vi "Dust_Source_Control.vi"(7 "error in":errorcluster) -> (0 "error out":errorcluster)   [LabVIEW 2015]
doc: "This VI specifies the properties of the pulse used for running the dust source. When program is stopped, the voltage is incrementally reduced to zero to avoid quick drops."
uses:
  Controls/dust_source_control.ctl
  Controls/XYVoltageFGV.ctl
  <vilib>/Utility/miscctls.llb/LVPointTypeDef.ctl
  <vilib>/Utility/error.llb/DialogType.ctl
  <vilib>/Utility/miscctls.llb/LVMinMaxIncTypeDef.ctl
  <vilib>/Utility/miscctls.llb/LVRangeTypeDef.ctl
  <vilib>/DAQmx/read.llb/DAQmx Read (Analog 1D Wfm NChan NSamp).vi
  <vilib>/Analysis/baseanly.llb/Mean (DBL).vi
  <vilib>/DAQmx/write.llb/DAQmx Write (Analog 1D Wfm NChan NSamp).vi
  <vilib>/DAQmx/read.llb/DAQmx Read (Counter U32 1Chan 1Samp).vi
  <vilib>/DAQmx/create/channels.llb/DAQmx Create Channel (AI-Voltage-Basic).vi
  <vilib>/DAQmx/configure/timing.llb/DAQmx Timing (Sample Clock).vi
  <vilib>/DAQmx/miscellaneous.llb/DAQmx Fill In Error Info.vi
  <vilib>/measure/mascope.llb/Amplitude and Levels 1 chan.vi
  <vilib>/DAQmx/create/channels.llb/DAQmx Create Channel (AO-Voltage-Basic).vi
  Global Variables/throttle.vi
  <userlib>/_OpenG.lib/comparison/comparison.llb/Boolean Changed__ogtk.vi
  Global Variables/throttle from query.vi
  <userlib>/_OpenG.lib/comparison/comparison.llb/DBL Changed__ogtk.vi
  Sub-Polymorphic/post_run_times.vi
  <vilib>/DAQmx/create/channels.llb/DAQmx Create Channel (CI-Count Edges).vi
  Sub-Polymorphic/update_counter_entry_big.vi
  Sub-Polymorphic/post_dust_source.vi
  <vilib>/addons/database/_DB Variant To Data/Database Variant To Data.xnode
  <resource>/objmgr/daqmx.rc
  <vilib>/measure/NI_MAPro.lvlib
  <vilib>/Analysis/NI_AALBase.lvlib
panel:
  out "Einzel and Steering":T1
  out "Y Vs":dbl[](array[numeric])
  out "X Vs":dbl[](array[numeric])
  out "Einzel Vs":dbl[](array[numeric])
  out "Old Einzel":dbl min=0.0 max=10.0 step=0.01 format="%.2g"
  out "Rate Data":dbl[][][](array[numeric])
  out "Freq. Before Throttle":dbl
  out "On/Off":bool
  out "Finished":bool=TRUE
  out "Output waveform":waveform(dbl)={"t0"=timestamp(0 s since 1904-01-01), "dt"=4e-06, "Y"=array[50000 elements]}
  out "Input waveform":waveform(dbl)={"t0"=timestamp(3437998856.0330505 s since 1904-01-01), "dt"=0.00019999999999999998, "Y"=array[1000 elements], "attributes"=variant("NI_ChannelName"=variant(string "Dev5/ai20"), "NI_UnitDescription"=variant(string "Volts"))}
  out "output cluster":T2={"Integer Timestamp"=0, "Einzel Voltage"=0.0, "Needle Voltage"=0.0, "Frequency"=1.0, "Width (ms) : 0.1 "=0.1, "Desired Amplitude (V)"=0.0, "X Voltage"=0.0, "Y Voltage"=0.0, "Settings ID"="", "ID#"=0} {"Needle Voltage" min=0.0 max=10.0 step=0.01 format="%.2g"; "Y Voltage" min=0.0 max=9.0 step=0.01 format="%.2g"; "X Voltage" min=0.0 max=9.0 step=0.01 format="%.2g"; "Einzel Voltage" min=0.0 max=10.0 step=0.01 format="%.2g"; "Desired Amplitude (V)" min=0.0 max=10.0 step=0.01 format="%5.2f"; "Width (ms) : 0.1" min=0.05 max=5.0 step=0.01 format="%6.2f"; "Frequency" min=1.0 max=100.0 step=0.01 format="%.1f"}
  in  "Tab Control":T3(tab)
  out "Current":dbl format="%.2f"
  out "Actual output width (ms)":dbl caption="Output Width (ms)" format="%.2f"
  out "Actual output Frequency":dbl caption="Output  Freq.(hz)" format="%.2f"
  in  "Width (ms) : 0.1":dbl=0.1 caption="Width (ms)" min=0.0 max=5.0 step=0.01 format="%6.2f"
  out "Tube Drive":dbl=0.0012999050305587314 format="%.2f"
  in  "Desired Amplitude (V)":dbl caption="Amplitude (V)" min=0.0 max=10.0 step=0.01 format="%5.2f"
  out "Actual output Amplitude (V)":dbl caption="Output Amp. (V)" format="%.2f"
  in  "Frequency":dbl=1.0 caption="Freq. (Hz)" min=0.0 max=30.0 step=0.01 format="%.1f"
  in  "Things to Scan":cluster{"Einzel":bool, "X":bool, "Y":bool}={"Einzel"=TRUE, "X"=TRUE, "Y"=TRUE}
  in  "Ein. Range":dbl[](array[numeric])=[0.0, 10.0] min=0.0 max=10.0 step=0.05 format="%#.2g"
  out "Steps to go":i32
  out "Num Steps":i16
  in  "# of Steps":i16[](array[numeric])=[5, 5, 5] min=0 max=10 step=1
  in  "Y Range":dbl[](array[numeric])=[-2.5, 2.5] min=-2.5 max=2.5 step=0.05 format="%#.2g"
  in  "X Range":dbl[](array[numeric])=[-2.5, 2.5] min=-2.5 max=2.5 step=0.05 format="%#.2g"
  in  "Calibrate XY":bool
  in  "Abort Change":bool
  out "Actual Needle (kV)":dbl=-1.1093266413053247 caption="Actual Einzel (V)" format="%.2f"
  out "Actual Needle Output (V)":dbl caption="Actual Einzel (V)" format="%.2f"
  in  "Needle Voltage":dbl min=0.0 max=10.0 step=0.01 format="%.2g"
  out "Actual Steerer Y (kV)":dbl=-0.02640654867851852 caption="Actual Einzel (V)" format="%.2f"
  out "Actual Y Output (V)":dbl=4.5 caption="Actual Einzel (V)" format="%.2f"
  in  "Y Voltage":dbl min=-2.5 max=2.5 step=0.01 format="%.2g"
  out "Actual Steerer X (kV)":dbl=-0.07767573560151271 caption="Actual Einzel (V)" format="%.2f"
  out "Actual X Output (V)":dbl=4.5 caption="Actual Einzel (V)" format="%.2f"
  in  "X Voltage":dbl min=-2.5 max=2.5 step=0.01 format="%.2g"
  out "Actual Einzel (kV)":dbl=-1.1709848579608468 caption="Actual Einzel (V)" format="%.2f"
  out "Actual Einzel Output (V)":dbl caption="Actual Einzel (V)" format="%.2f"
  in  "Einzel Voltage":dbl min=0.0 max=10.0 step=0.01 format="%.2g"
  in  "Save Settings?":bool
  in  "Settings ID":string
  out "CONTROLS":waveform(dbl)[](graph)=[{"t0"=timestamp(0 s since 1904-01-01), "dt"=4e-06, "Y"=array[50000 elements]}, {"t0"=timestamp(3437998856.0330505 s since 1904-01-01), "dt"=0.00019999999999999998, "Y"=array[1000 elements], "attributes"=variant("NI_ChannelName"=variant(string "Dev5/ai20"), "NI_UnitDescription"=variant(string "Volts"))}]
  in  "Retrieve Settings":bool
  out "Det2/Det1":dbl
  out "Det3/Det1":dbl
  out "PSU/Det3":dbl
  out "PSU/Det2":dbl
  out "First detector since\nlast source change:":i64
  out "Third detector since\nlast source change:":i64
  out "Source Efficiency":dbl
  out "Det1 Rate":dbl
  out "PSU Rate":dbl
  out "Det3 Rate":dbl
  in  "Cycles to Avg.":i32=10
  out "Hours Run":dbl
  in  "Alarm Threshold":dbl=15.0
  in  "Y Slice":dbl(slide) min=-2.5 max=2.5 step=1.25 scale=-2.5..2.5
  in  "X Slice":dbl(slide) min=-2.5 max=2.5 step=1.25 scale=-2.5..2.5
  in  "Einzel Slice":dbl(slide) min=0.0 max=10.0 step=2.5 scale=0.0..10.0
  out "Y Slice Data":dbl[][](graph)
  out "X Slice Data":dbl[][](graph)
  out "Einzel Slice Data":dbl[][](graph)
  in  "Maximums":cluster{"Width":dbl, "Freq.":dbl}
  out "Testing":bool
  in  "Physical Output Channels":tag="Dev4/ao19, Dev4/ao9, Dev4/ao11:12, Dev4/ao16"
  in  "Physical Input Channels":tag="Dev5/ai19:23"
  out "Execution Number:":i32=341
  in  "Cal Test?":bool
  in  "Counters On/Off":bool=TRUE
  in  "Reset Counters":bool
  in  "Det1":tag="Dev5/ctr0"
  in  "Det2":tag="Dev5/ctr1"
  in  "Det3":tag="Dev4/ctr0"
  in  "PSU":tag="Dev4/ctr1"
  out "PSU":u32
  out "Det3":u32
  out "Det2":u32
  out "Det1":u32
  out "error?":bool
  out "Actual Sample Clock Rate":dbl=250000.0 format="%.2f"
  in  "stop":bool
  # "Dust Source Control"
  # "Hold Down to\nStop Changes"
  # "Tube Drive (Ao0, Ai4)"
  # "E"
  # "x"
  # "y"
  # "Needle Control (Ao4, Ai0)"
  # "Steerer Y Control (Ao3, Ai3)"
  # "Steerer X Control (Ao2, Ai2)"
  # "Einzel Lens (Ao1, Ai1)"
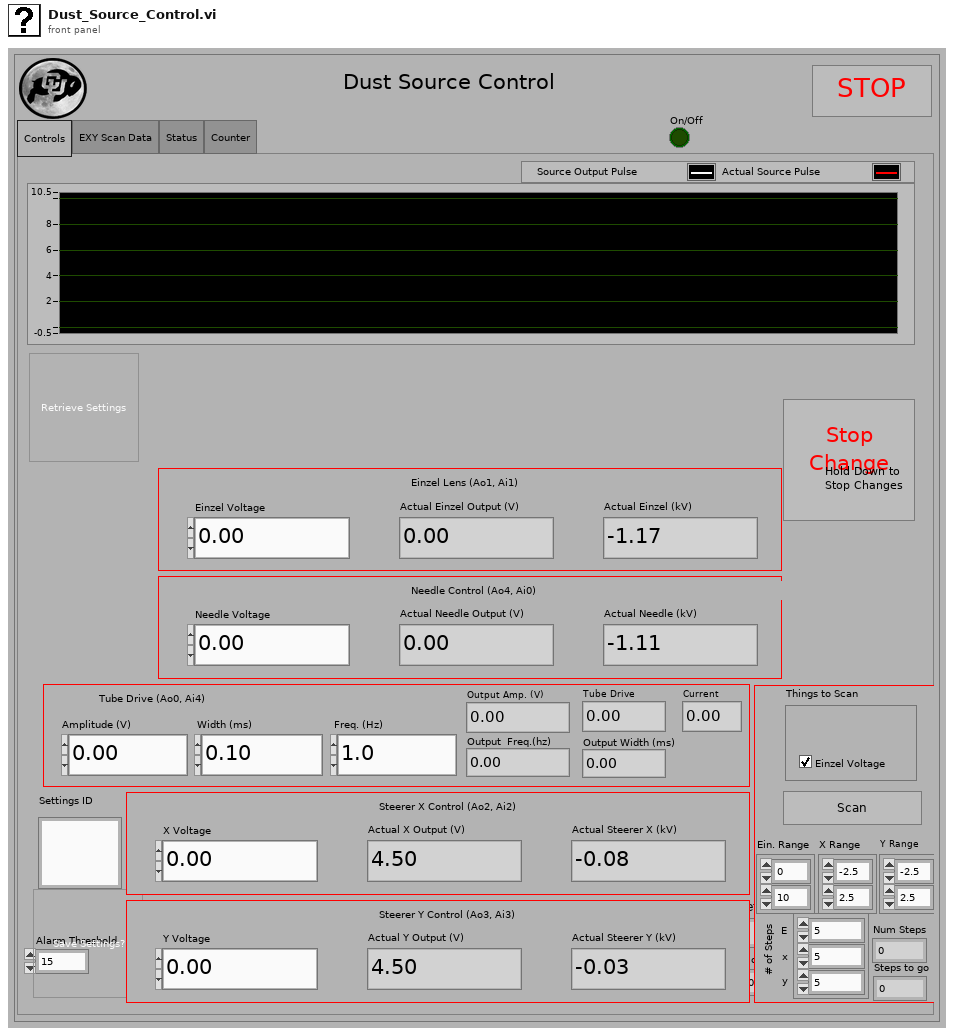
[diagram p1: front panel]
types:
  T1 = cluster{"Einzel Voltage":dbl, "X Voltage":dbl, "Y Voltage":dbl}
  T2 = typedef "dust_source_control.ctl" = cluster{"Integer Timestamp":u64, "Einzel Voltage":dbl, "Needle Voltage":dbl, "Frequency":dbl, "Width (ms) : 0.1 ":dbl, "Desired Amplitude (V)":dbl, "X Voltage":dbl, "Y Voltage":dbl, "Settings ID":string, "ID#":i32}
  T3 = enum32{"Controls", "EXY Scan Data", "Status", "Counter"}
  T4 = typedef "LVPointTypeDef.ctl" = cluster{"Horizontal":i16, "Vertical":i16}
  T5 = typedef "XYVoltageFGV.ctl" = u16
  T6 = enum8{"Enabled", "Disabled", "Disabled and Grayed Out"}
  T7 = typedef "DialogType.ctl" = u16
  T8 = typedef "LVRangeTypeDef.ctl" = cluster{"Minimum":dbl, "Maximum":dbl, "Increment":dbl, "Minor Increment":dbl, "Start":dbl}
  T9 = typedef "LVMinMaxIncTypeDef.ctl" = cluster{"Minimum":dbl, "Maximum":dbl, "Increment":dbl}
  T10 = cluster{"data":u32, "data":u32, "data":u32, "data":u32}
  T11 = cluster{"Minimum":dbl, dbl, "Increment":dbl, "Minor Increment":dbl, "Start":dbl}
  T12 = cluster{"Integer Time":i64, "Integer Time":i64, "Experiment ID":i64}
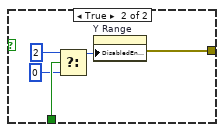
[diagram p2: hidden frame]
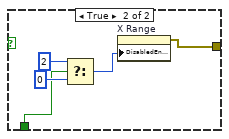
[diagram p3: hidden frame]
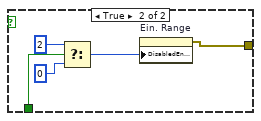
[diagram p4: hidden frame]
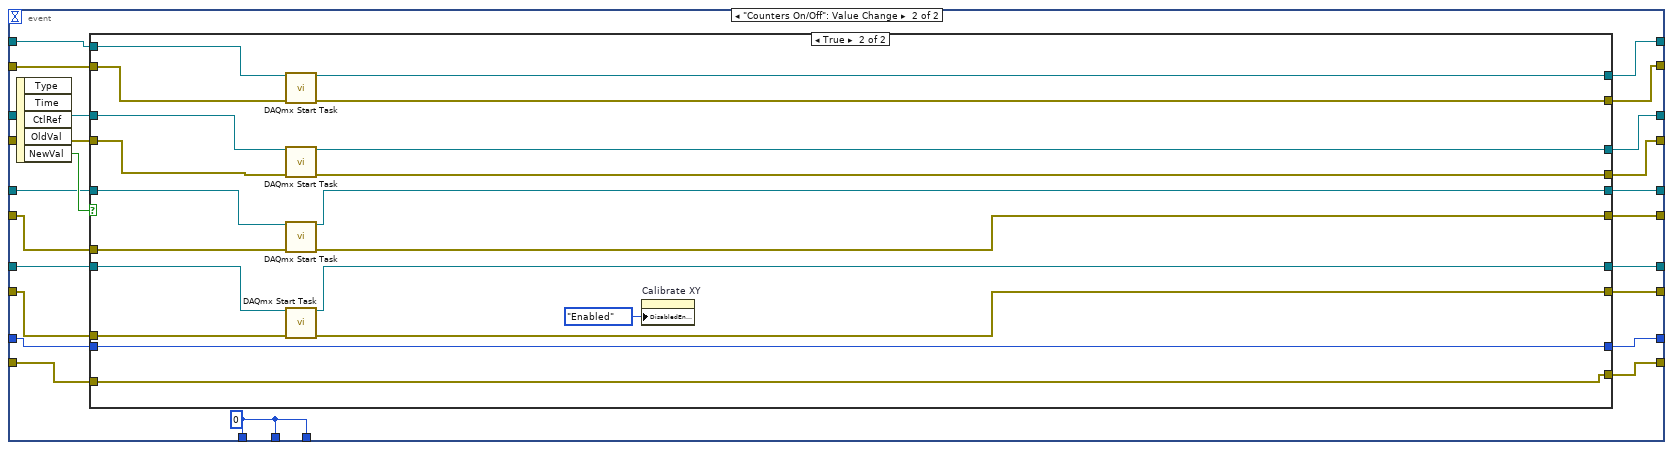
[diagram p8: hidden frame]
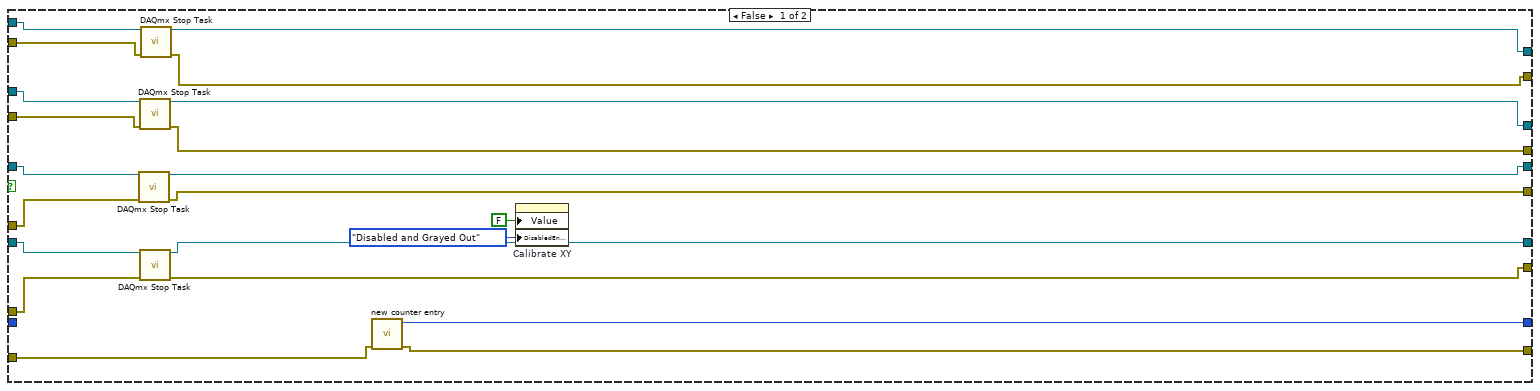
[diagram p9: hidden frame]
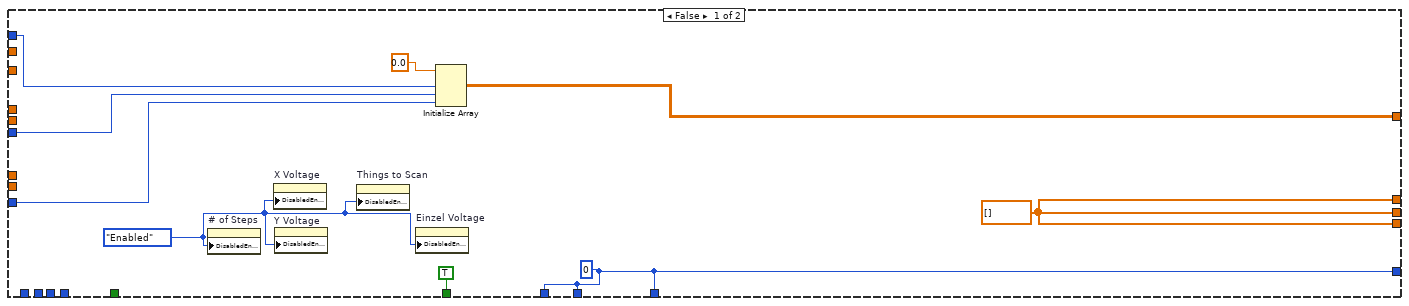
[diagram p10: hidden frame]
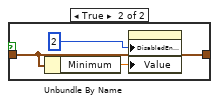
[diagram p11: hidden frame]
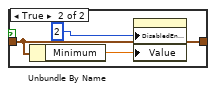
[diagram p12: hidden frame]
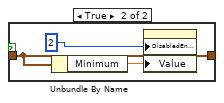
[diagram p13: hidden frame]
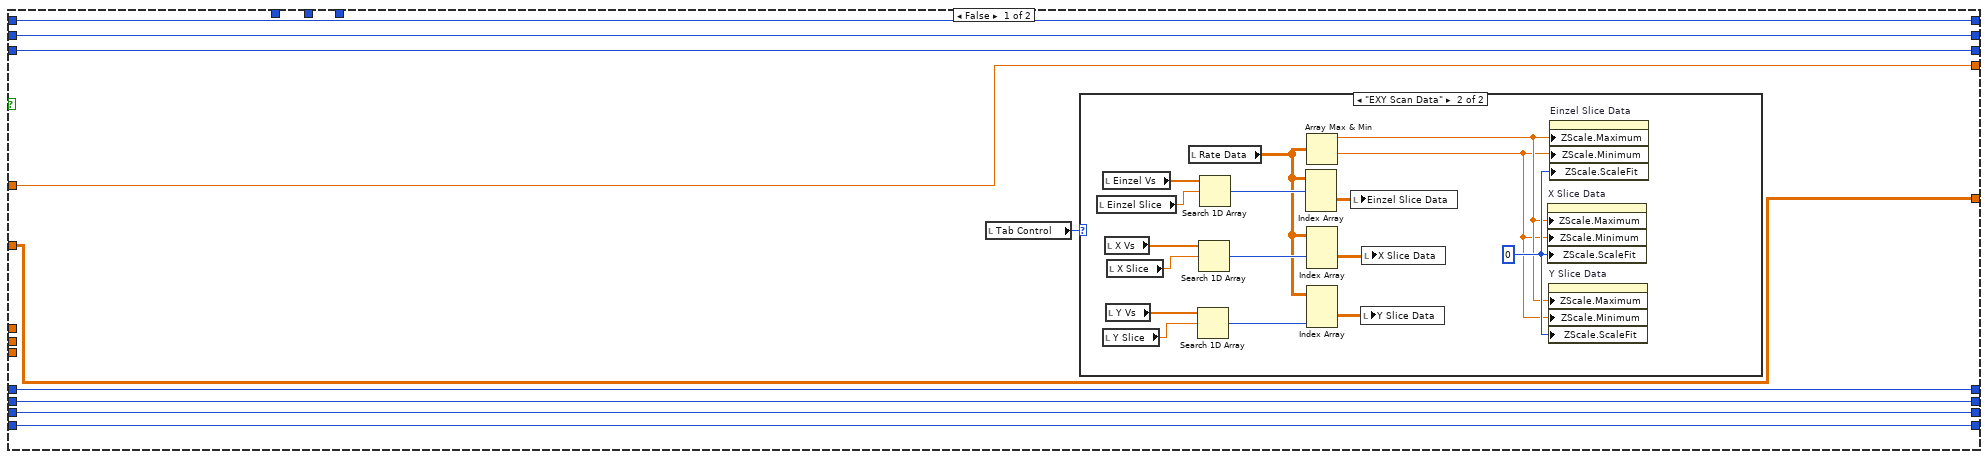
[diagram p15: hidden frame]
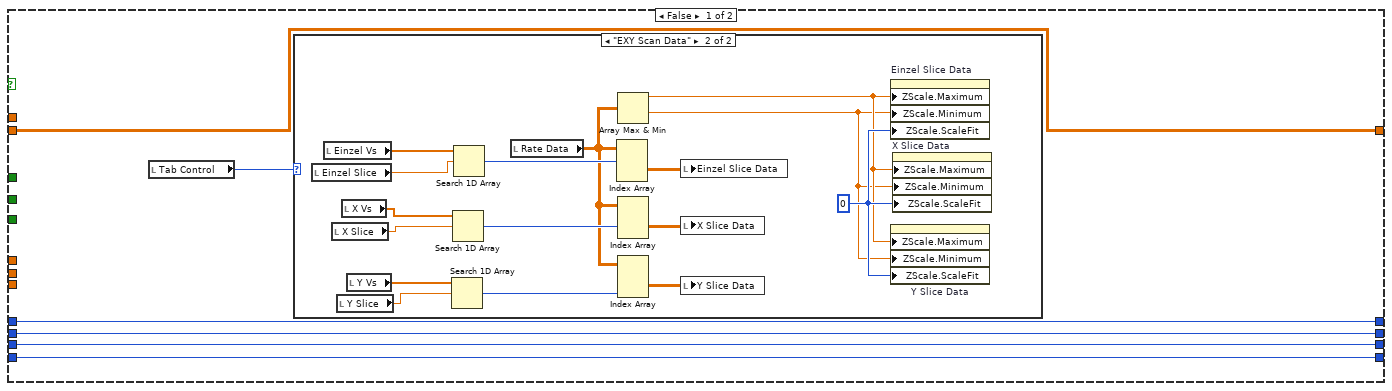
[diagram p17: hidden frame]
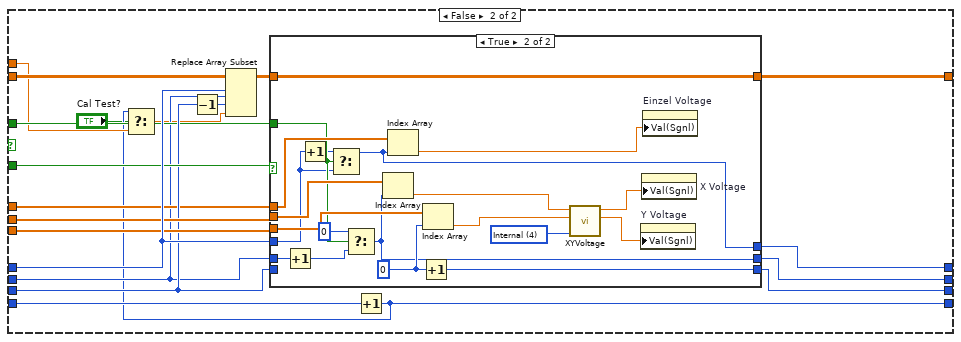
[diagram p20: hidden frame]
diagram:
  w31 = 0
  w40 = T5 4 items=["Get", "Set X", "Set Y", "Set XY", "Internal"] ("Ring")
  w18 = T6."Enabled" ("Disabled")
  w19 = FALSE ("Retrieve Settings")
  w3 = 0.0 ("Actual Output (V)")
  w41 = FALSE ("Shutdown")
  # "Play Startup Sound"
  # "Initialization stuff"
  n1 = call "DB_Query.vi"("error in (no error)"="error in", "Parameterized Query"="SELECT\n  dust_name,\n  dust_type.dust_type,\n  batch_no\nFROM\n  dust_type\n    INNER JOIN\n  dust_info\n    ON\n      dust_type.id_dust_type = dust_info.dust_type\nORDER BY\n  dust_info.integer_timestamp DESC\nLIMIT 1;" ("SQL query")) -> ("error out"=w5:errorcluster, "Results"=w4:variant[][])  [unwired: 7 in, 1 out]
  n2 = control-ref of="This VI"() -> (w17:refnum<vi>)
  n3 = Index Array(array=w4) -> (element=w38:variant[])  [unwired: 2 in]
  n4 = Index Array(array=w38) -> (element #1=w37:variant, element #2=w34:variant, element #3=w33:variant)  [unwired: 3 in]
  n5 = property class="VI"(reference=w17, error in="error in") -> (error out=w16:errorcluster, "Panel"=w15:refnum<vi>)  [unwired: 1 out]
  n6 = xnode "Database Variant To Data"("database variant"=w37, "error in (no error)"=w5, "type"="") -> ("data"=w29:string, "error out"=w36:errorcluster)
  n7 = property class="Pnl"(reference=w15, error in=w16) -> (error out=w14:errorcluster, "Panes[]"=w13:refnum<vi>[])  [unwired: 1 out]
  n8 = call "Play_Sound.vi"("Sound Type"=4) -> ()  [unwired: 1 in, 1 out]
  n9 = call "XYVoltage.vi"("X Voltage"=w3, "Y Voltage"=w3, "Ring"=w40) -> ("X Voltage 2"=w20:dbl)  [unwired: 5 in, 2 out]
  n10 = String To IP() -> (0:w25:u32)  [unwired: 1 in]
  n11 = xnode "Database Variant To Data"("database variant"=w34, "error in (no error)"=w36, "type"=w31) -> ("data"=w28:i32, "error out"=w35:errorcluster)
  n12 = local write "Counters On/Off"(TRUE ("Counters On/Off")) -> ()
  n13 = IP To String(2:w25) -> (0:w24:string)  [unwired: 1 in]
  n14 = local write "Maximums"(cluster{"Width":dbl, "Freq.":dbl} {"Width"=5.0, "Freq."=30.0} ("Maximums")) -> ()
  n15 = local write "Actual Einzel Output (V)"(w3) -> ()
  n16 = local write "Actual output Amplitude (V)"(w3) -> ()
  n17 = local write "Einzel Voltage"(w3) -> ()
  n18 = local write "Actual X Output (V)"(w3) -> ()
  n19 = local write "Actual Needle Output (V)"(w3) -> ()
  n20 = local write "Needle Voltage"(w3) -> ()
  n21 = local write "Actual output Amplitude (V)"(w3) -> ()
  n22 = local write "Desired Amplitude (V)"(w3) -> ()
  n23 = local write "Einzel Voltage"(w3) -> ()
  n24 = local write "Actual Einzel Output (V)"(w3) -> ()
  n25 = local write "Actual X Output (V)"(w3) -> ()
  n26 = local write "Actual Y Output (V)"(w3) -> ()
  n27 = local write "Frequency"(w3) -> ()
  n28 = local write "Y Voltage"(w20) -> ()
  n29 = local write "Width (ms) : 0.1"(w3) -> ()
  n30 = local write "Finished"(FALSE ("Finished")) -> ()
  n31 = local write "Retrieve Settings"(w19) -> ()
  n32 = local write "Save Settings?"(w19) -> ()
  n33 = local write "X Voltage"(w20) -> ()
  n34 = local write "stop"(w41) -> ()
  n35 = local write "Cal Test?"(w19) -> ()
  n36 = local write "Old Einzel"(w20) -> ()
  n37 = local write "Calibrate XY"(w41) -> ()
  n38 = Index Array(array=w13, index=0) -> (element=w11:refnum<vi>)
  n39 = property on="Things to Scan" class="Clust (strict)"("DisabledEnum"=w18) -> ()  [unwired: 2 in, 2 out]
  n40 = property on="Ein. Range" class="Arr (strict)"("DisabledEnum"=w18) -> ()  [unwired: 2 in, 2 out]
  n41 = property on="Y Range" class="Arr (strict)"("DisabledEnum"=w18) -> ()  [unwired: 2 in, 2 out]
  n42 = property on="# of Steps" class="Arr (strict)"("DisabledEnum"=w18) -> ()  [unwired: 2 in, 2 out]
  n43 = property on="Calibrate XY" class="Bool (strict)"("DisabledEnum"=w18) -> ()  [unwired: 2 in, 2 out]
  n44 = property on="Einzel Voltage" class="DigNum (strict)"("DisabledEnum"=w18) -> ()  [unwired: 2 in, 2 out]
  n45 = property on="Y Voltage" class="DigNum (strict)"("DisabledEnum"=w18) -> ()  [unwired: 2 in, 2 out]
  n46 = property on="X Voltage" class="DigNum (strict)"("DisabledEnum"=w18) -> ()  [unwired: 2 in, 2 out]
  n47 = property on="X Range" class="Arr (strict)"("DisabledEnum"=w18) -> ()  [unwired: 2 in, 2 out]
  n48 = Not Equal?(x=w24, y="Schrödinger") -> (x != y?=w22:bool)
  "Testing" <- w22
  n49 = xnode "Database Variant To Data"("database variant"=w33, "error in (no error)"=w35, "type"=w31) -> ("data"=w27:i32, "error out"=w2:errorcluster)
  n50 = property class="Pane"(reference=w11, error in=w14, "Origin"=T4 {"Horizontal"=0, "Vertical"=0}) -> (error out=w9:errorcluster)  [unwired: 1 out]
  n51 = Format Into String(format string="DT: %s-%0.0g-%0.0g", w29, w28, w27) -> (resulting string=w26:string)  [unwired: 2 in, 1 out]
  n52 = Merge Errors(w9, w2) -> (w8:errorcluster)
  n53 = case shown="No Error" w8 {
    selector: w8 -> [w63 w2287]
    tunnel: [w45 w2287] -> w43
    tunnel: w26 -> [w51 _]
    tunnel: w22 -> [w50 _]
    frame No Error {
      w54 = 0.0 ("Width (ms) : 3.5")
      w49 = dbl[] []
      w47 = 0
      w73 = 10252 items=["Overwrite Unread Samples"=10252, "Do Not Overwrite Unread Samples"=10159] ("OverWrite")
      w74 = TRUE ("ReadAllAvailSamp")
      w46 = u32 0 ("data")
      w44 = 50000.0 ("Size (Samples)")
      w137 = 10097 items=["Allow Regeneration"=10097, "Do Not Allow Regeneration"=10158] ("RegenMode")
      w142 = T7 3 items=["no dialog", "OK message", "continue or stop message", "OK message + warnings", "continue/stop + warnings"] ("type of dialog (OK msg:1)")
      w146 = 10123 items=["Finite Samples"=10178, "Continuous Samples"=10123] ("sample mode")
      # "Plot updating loop"
      # "Output channel initilization"
      n54 = local read "output cluster"() -> (w126:T2)
      n55 = while {
        shift-right: [w888] -> w82
        shift-left: w63 -> [w887]
        shift-right: [w891] -> _
        shift-left: w126 -> [w890]
        tunnel: w51 -> [w885]
        tunnel: w50 -> [w883]
        stop <- w886 stop-if-true
        n56 = Select(t=1000, s=w883, f=300000) -> (s? t:f=w884:i32)
        n57 = event shown="[0] Timeout" {
          selector: _ -> [_ _ _ _]
          dyn-events: _ -> [_ _ _ _]
          timeout: w884 -> [_ _ _ _]
          tunnel: [w917 w992 w1023 w1060] -> w891
          tunnel: w890 -> [w916 w992 _ _]
          tunnel: [w911 w993 w1007 w1062] -> w888
          tunnel: w887 -> [w912 w993 w1005 w1061]
          tunnel: [w913 w989 w1020 _] -> w886
          tunnel: w885 -> [w910 _ w997 _]
          event Timeout {
            n58 = event-data() -> ()  [unwired: 1 in, 2 out]
            n59 = local read "output cluster"() -> (w917:T2)
            n60 = Unbundle By Name(w917) -> ("Einzel Voltage"=w908:dbl, "Needle Voltage"=w907:dbl, "Frequency"=w906:dbl, "Width (ms) : 0.1"=w905:dbl, "Desired Amplitude (V)"=w904:dbl, "X Voltage"=w903:dbl, "Y Voltage"=w902:dbl)
            n61 = Unbundle By Name(w916) -> ("Einzel Voltage"=w896:dbl, "Needle Voltage"=w895:dbl, "Frequency"=w897:dbl, "Width (ms) : 0.1"=w901:dbl, "Desired Amplitude (V)"=w900:dbl, "X Voltage"=w899:dbl, "Y Voltage"=w898:dbl)
            n62 = Build Array(w908, w907, w906, w905, w904, w903, w902) -> (w893:dbl[])
            n63 = Build Array(w896, w895, w897, w901, w900, w899, w898) -> (w894:dbl[])
            n64 = Equal?(x=w893, y=w894) -> (x = y?=w909:bool[])
            n65 = And Array Elements(Boolean array=w909) -> (logical AND=w892:bool)
            n66 = case shown="False" w892 {
              tunnel: w912 -> [w923 w988]
              tunnel: [w933 w988] -> w911
              tunnel: w910 -> [w928 _]
              frame False {
                w918 = 0 ("index (row)")
                n67 = call "DB_Query.vi"("error in (no error)"=w923, "Parameterized Query"="SELECT\n  high_voltage\nFROM\n  pelletron_data\nORDER BY\n  id_pelletron_data DESC\nLIMIT 1; " ("SQL query")) -> ("error out"=w924:errorcluster, "Results"=w925:variant[][])  [unwired: 7 in, 1 out]
                n68 = Get Date/Time In Seconds() -> (seconds since 1Jan1904=w949:timestamp)
                n69 = local read "output cluster"() -> (w935:T2)
                n70 = Index Array(array=w925, index (row)=w918, index (col)=w918) -> (element=w932:variant)
                n71 = xnode "Database Variant To Data"("database variant"=w932, "error in (no error)"=w924, "type"=0.0 ("input 1")) -> ("data"=w930:dbl, "error out"=w922:errorcluster)
                n72 = Unbundle By Name(w935) -> ("Einzel Voltage"=w948:dbl, "Needle Voltage"=w947:dbl, "Frequency"=w941:dbl, "Width (ms) : 0.1"=w940:dbl, "Desired Amplitude (V)"=w946:dbl, "X Voltage"=w944:dbl, "Y Voltage"=w943:dbl)
                n73 = Format Date/Time String(seconds (now)=w949) -> (date/time string=w921:string)  [unwired: 2 in]
                n74 = Format Into String(format string=" (%s; HV: %0.1f; Time: %s)", initial string="Automatic Update", w928, w930, w921) -> (resulting string=w920:string)  [unwired: 1 in, 1 out]
                n75 = call "LV_to_int_time.vi"("error in (no error)"=w922, "Time Stamp"=w949) -> ("error out"=w950:errorcluster, "Integer Time"=w951:i64)  [unwired: 7 in]
                n76 = Bundle By Name(cluster=w935, "Einzel Voltage"=w948, "Needle Voltage"=w947, "Frequency"=w941, "Width (ms) : 0.1"=w940, "Desired Amplitude (V)"=w946, "X Voltage"=w944, "Y Voltage"=w943, "Integer Timestamp"=w951, "Settings ID"=w920) -> (w936:T2)
                n77 = Build Array(w947, w946) -> (w945:dbl[])
                n78 = Less Or Equal?(x=w940, y=0.01) -> (x <= y?=w934:bool)
                n79 = Less?(x=w945, y=0.1) -> (x < y?=w938:bool[])
                n80 = Build Array (concatenate)(w938, w934) -> (w937:bool[])
                n81 = Or Array Elements(Boolean array=w937) -> (logical OR=w927:bool)
                n82 = case shown="False" w927 {
                  tunnel: w936 -> [w984 _]
                  tunnel: [w986 w987] -> w933
                  tunnel: w950 -> [w985 w987]
                  frame False {
                    n83 = call-poly "post_to_db.vi"("error in (no error)"=w985, "Dust control settings"=w984) -> ("error out"=w986:errorcluster)  [unwired: 9 in]
                  }
                  frame True {
                  }
                }
              }
              frame True {
              }
            }
            n84 = local read "error?"() -> (w914:bool)
            n85 = local read "stop"() -> (w915:bool)
            n86 = Or(x=w915, y=w914) -> (x .or. y?=w913:bool)
          }
          event "stop": Value Change {
            n87 = event-data() -> ()  [unwired: 1 in, 5 out]
            n88 = local read "stop"() -> (w991:bool)
            n89 = local read "error?"() -> (w990:bool)
            n90 = Or(x=w991, y=w990) -> (x .or. y?=w989:bool)
          }
          event "Save Settings?": Value Change {
            w1002 = 0 ("index (row)")
            n91 = event-data() -> ()  [unwired: 1 in, 5 out]
            n92 = local read "output cluster"() -> (w1023:T2)
            n93 = call "DB_Query.vi"("error in (no error)"=w1005, "Parameterized Query"="SELECT\n  high_voltage\nFROM\n  pelletron_data\nORDER BY\n  id_pelletron_data DESC\nLIMIT 1;" ("SQL query")) -> ("error out"=w1001:errorcluster, "Results"=w1003:variant[][])  [unwired: 7 in, 1 out]
            n94 = Get Date/Time In Seconds() -> (seconds since 1Jan1904=w1019:timestamp)
            n95 = Index Array(array=w1003, index (row)=w1002, index (col)=w1002) -> (element=w1010:variant)
            n96 = Format Date/Time String(time format string (%c)=" time: %c" ("Settings ID"), seconds (now)=w1019) -> (date/time string=w995:string)  [unwired: 1 in]
            n97 = Unbundle By Name(w1023) -> ("Einzel Voltage"=w1018:dbl, "Needle Voltage"=w1017:dbl, "Frequency"=w1016:dbl, "Width (ms) : 0.1"=w1015:dbl, "Desired Amplitude (V)"=w1014:dbl, "X Voltage"=w1013:dbl, "Y Voltage"=w1012:dbl)
            n98 = xnode "Database Variant To Data"("database variant"=w1010, "error in (no error)"=w1001, "type"=0.0 ("input 1")) -> ("data"=w998:dbl, "error out"=w1000:errorcluster)
            n99 = call "LV_to_int_time.vi"("error in (no error)"=w1005, "Time Stamp"=w1019) -> ("error out"=w1021:errorcluster, "Integer Time"=w1022:i64)  [unwired: 7 in]
            n100 = Format Into String(format string=" (%s; HV: %0.1f; Time: %s)", initial string="Settings ID", w997, w998, w995) -> (resulting string=w994:string)  [unwired: 1 in, 1 out]
            n101 = Bundle By Name(cluster=w1023, "Einzel Voltage"=w1018, "Needle Voltage"=w1017, "Frequency"=w1016, "Width (ms) : 0.1"=w1015, "Desired Amplitude (V)"=w1014, "X Voltage"=w1013, "Y Voltage"=w1012, "Integer Timestamp"=w1022, "Settings ID"=w994) -> (w1006:T2)
            n102 = call-poly "post_to_db.vi"("error in (no error)"=w1021, "Dust control settings"=w1006) -> ("error out"=w1008:errorcluster)  [unwired: 9 in]
            n103 = Merge Errors(w1008, w1000) -> (w1007:errorcluster)
            n104 = flat-sequence {
              tunnel: [w1057] -> w1020
              frame #0 {
                n105 = Wait (ms)(milliseconds to wait=u32 100) -> ()  [unwired: 1 out]
              }
              frame #1 {
                w1057 = FALSE
                n106 = local write "Save Settings?"(w1057) -> ()
              }
            }
          }
          event "Retrieve Settings": Value Change {
            n107 = event-data() -> ()  [unwired: 1 in, 5 out]
            n108 = local write "Retrieve Settings"(FALSE) -> ()
            n109 = call "Query_source_settings_menu.vi"("error in (no error)"=w1061) -> ("error out"=w1059:errorcluster, "Cancelled?"=w1058:bool, "Output cluster"=w1060:T2)  [unwired: 8 in]
            n110 = Unbundle By Name(w1060) -> ("Einzel Voltage"=w1070:dbl, "Needle Voltage"=w1069:dbl, "Frequency"=w1068:dbl, "Width (ms) : 0.1"=w1067:dbl, "Desired Amplitude (V)"=w1066:dbl, "X Voltage"=w1065:dbl, "Y Voltage"=w1064:dbl)
            n111 = case shown="False" w1058 {
              tunnel: w1070 -> [w1083 _]
              tunnel: w1059 -> [w1107 w1215]
              tunnel: w1069 -> [w1080 _]
              tunnel: w1068 -> [w1074 _]
              tunnel: w1067 -> [w1077 _]
              tunnel: w1066 -> [w1073 _]
              tunnel: w1065 -> [w1106 _]
              tunnel: w1064 -> [w1090 _]
              tunnel: [w1084 w1215] -> w1062
              frame False {
                n112 = flat-sequence {
                  tunnel: w1107 -> [w1109]
                  tunnel: [w1108] -> w1105
                  tunnel: w1106 -> [w1110]
                  tunnel: [w1110] -> w1104
                  tunnel: w1105 -> [w1112]
                  tunnel: [w1112] -> w1103
                  tunnel: w1104 -> [w1111]
                  tunnel: [w1111] -> w1102
                  tunnel: w1103 -> [w1115]
                  tunnel: [w1114] -> w1101
                  tunnel: w1102 -> [w1116]
                  tunnel: w1101 -> [w1130]
                  tunnel: [w1131] -> w1089
                  tunnel: w1090 -> [w1129]
                  tunnel: [w1129] -> w1085
                  tunnel: w1089 -> [w1134]
                  tunnel: [w1134] -> w1088
                  tunnel: [w1132] -> w1086
                  tunnel: w1085 -> [w1132]
                  tunnel: w1088 -> [w1137]
                  tunnel: [w1136] -> w1087
                  tunnel: w1086 -> [w1135]
                  tunnel: w1087 -> [w1151]
                  tunnel: [w1152] -> w1100
                  tunnel: w1083 -> [w1150]
                  tunnel: [w1150] -> w1082
                  tunnel: w1100 -> [w1154]
                  tunnel: [w1154] -> w1099
                  tunnel: w1082 -> [w1153]
                  tunnel: [w1153] -> w1081
                  tunnel: w1099 -> [w1157]
                  tunnel: [w1158] -> w1098
                  tunnel: w1081 -> [w1156]
                  tunnel: w1098 -> [w1168]
                  tunnel: [w1169] -> w1097
                  tunnel: w1080 -> [w1167]
                  tunnel: [w1167] -> w1078
                  tunnel: [w1171] -> w1096
                  tunnel: w1097 -> [w1171]
                  tunnel: [w1170] -> w1079
                  tunnel: w1078 -> [w1170]
                  tunnel: w1096 -> [w1174]
                  tunnel: [w1175] -> w1095
                  tunnel: w1079 -> [w1173]
                  tunnel: w1095 -> [w1189]
                  tunnel: [w1188] -> w1094
                  tunnel: w1073 -> [w1187]
                  tunnel: [w1187] -> w1071
                  tunnel: w1094 -> [w1192]
                  tunnel: [w1193] -> w1093
                  tunnel: w1077 -> [w1191]
                  tunnel: [w1190] -> w1072
                  tunnel: w1071 -> [w1190]
                  tunnel: w1093 -> [w1196]
                  tunnel: [w1195] -> w1092
                  tunnel: [w1197] -> w1075
                  tunnel: w1074 -> [w1194]
                  tunnel: w1072 -> [w1197]
                  tunnel: w1092 -> [w1199]
                  tunnel: [w1199] -> w1091
                  tunnel: [w1198] -> w1076
                  tunnel: w1075 -> [w1198]
                  tunnel: w1091 -> [w1203]
                  tunnel: [w1202] -> w1084
                  tunnel: w1076 -> [w1201]
                  frame #0 {
                    n113 = property on="X Voltage" class="DigNum (strict)"(error in=w1109, "Val(Sgnl)"=w1110) -> (error out=w1108:errorcluster)  [unwired: 1 in, 1 out]
                  }
                  frame #1 {
                    n114 = Wait (ms)(milliseconds to wait=u32 100) -> ()  [unwired: 1 out]
                  }
                  frame #2 {
                    n115 = while {
                      tunnel: w1116 -> [w1124]
                      shift-right: [w1128] -> w1114
                      shift-left: w1115 -> [w1128]
                      stop <- w1122 stop-if-true
                      n116 = local read "Actual X Output (V)"() -> (w1117:dbl)
                      n117 = local read "stop"() -> (w1119:bool)
                      n118 = local read "Abort Change"() -> (w1120:bool)
                      n119 = call "scale xy steering.vi"("0 to 9 V input"=w1117) -> ("-2.5 to 2.5 V output"=w1118:dbl)  [unwired: 1 in, 1 out]
                      n120 = Subtract(x=w1124, y=w1118) -> (x-y=w1127:dbl)
                      n121 = Absolute Value(x=w1127) -> (abs(x)=w1126:dbl)
                      n122 = Or(x=w1119, y=w1120) -> (x .or. y?=w1121:bool)
                      n123 = Less?(x=w1126, y=0.1) -> (x < y?=w1123:bool)
                      n124 = Or(x=w1123, y=w1121) -> (x .or. y?=w1122:bool)
                    }
                  }
                  frame #3 {
                    n125 = property on="Y Voltage" class="DigNum (strict)"(error in=w1130, "Val(Sgnl)"=w1129) -> (error out=w1131:errorcluster)  [unwired: 1 in, 1 out]
                  }
                  frame #4 {
                    n126 = Wait (ms)(milliseconds to wait=u32 100) -> ()  [unwired: 1 out]
                  }
                  frame #5 {
                    n127 = while {
                      shift-right: [w1149] -> w1136
                      shift-left: w1137 -> [w1149]
                      tunnel: w1135 -> [w1140]
                      stop <- w1143 stop-if-true
                      n128 = local read "Actual Y Output (V)"() -> (w1139:dbl)
                      n129 = local read "Abort Change"() -> (w1142:bool)
                      n130 = local read "stop"() -> (w1141:bool)
                      n131 = call "scale xy steering.vi"("0 to 9 V input"=w1139) -> ("-2.5 to 2.5 V output"=w1138:dbl)  [unwired: 1 in, 1 out]
                      n132 = Subtract(x=w1140, y=w1138) -> (x-y=w1148:dbl)
                      n133 = Absolute Value(x=w1148) -> (abs(x)=w1147:dbl)
                      n134 = Or(x=w1142, y=w1141) -> (x .or. y?=w1144:bool)
                      n135 = Less?(x=w1147, y=0.1) -> (x < y?=w1146:bool)
                      n136 = Or(x=w1146, y=w1144) -> (x .or. y?=w1143:bool)
                    }
                  }
                  frame #6 {
                    n137 = property on="Einzel Voltage" class="DigNum (strict)"(error in=w1151, "Val(Sgnl)"=w1150) -> (error out=w1152:errorcluster)  [unwired: 1 in, 1 out]
                  }
                  frame #7 {
                    n138 = Wait (ms)(milliseconds to wait=u32 100) -> ()  [unwired: 1 out]
                  }
                  frame #8 {
                    n139 = while {
                      shift-right: [w1166] -> w1158
                      shift-left: w1157 -> [w1166]
                      tunnel: w1156 -> [w1159]
                      stop <- w1163 stop-if-true
                      n140 = local read "Actual Einzel Output (V)"() -> (w1164:dbl)
                      n141 = local read "Abort Change"() -> (w1162:bool)
                      n142 = local read "stop"() -> (w1160:bool)
                      n143 = Or(x=w1162, y=w1160) -> (x .or. y?=w1161:bool)
                      n144 = Equal?(x=w1164, y=w1159) -> (x = y?=w1165:bool)
                      n145 = Or(x=w1165, y=w1161) -> (x .or. y?=w1163:bool)
                    }
                  }
                  frame #9 {
                    n146 = property on="Needle Voltage" class="DigNum (strict)"(error in=w1168, "Val(Sgnl)"=w1167) -> (error out=w1169:errorcluster)  [unwired: 1 in, 1 out]
                  }
                  frame #10 {
                    n147 = Wait (ms)(milliseconds to wait=u32 100) -> ()  [unwired: 1 out]
                  }
                  frame #11 {
                    n148 = while {
                      shift-right: [w1186] -> w1175
                      shift-left: w1174 -> [w1186]
                      tunnel: w1173 -> [w1176]
                      stop <- w1180 stop-if-true
                      n149 = local read "Actual Needle Output (V)"() -> (w1182:dbl)
                      n150 = local read "stop"() -> (w1177:bool)
                      n151 = local read "Abort Change"() -> (w1179:bool)
                      n152 = Subtract(x=w1182, y=w1176) -> (x-y=w1185:dbl)
                      n153 = Absolute Value(x=w1185) -> (abs(x)=w1184:dbl)
                      n154 = Or(x=w1177, y=w1179) -> (x .or. y?=w1178:bool)
                      n155 = Less?(x=w1184, y=0.1) -> (x < y?=w1181:bool)
                      n156 = Or(x=w1178, y=w1181) -> (x .or. y?=w1180:bool)
                    }
                  }
                  frame #12 {
                    n157 = property on="Desired Amplitude (V)" class="DigNum (strict)"(error in=w1189, "Val(Sgnl)"=w1187) -> (error out=w1188:errorcluster)  [unwired: 1 in, 1 out]
                  }
                  frame #13 {
                    n158 = property on="Width (ms) : 0.1" class="DigNum (strict)"(error in=w1192, "Val(Sgnl)"=w1191) -> (error out=w1193:errorcluster)  [unwired: 1 in, 1 out]
                  }
                  frame #14 {
                    n159 = property on="Frequency" class="DigNum (strict)"(error in=w1196, "Val(Sgnl)"=w1194) -> (error out=w1195:errorcluster)  [unwired: 1 in, 1 out]
                  }
                  frame #15 {
                    n160 = Wait (ms)(milliseconds to wait=u32 100) -> ()  [unwired: 1 out]
                  }
                  frame #16 {
                    n161 = while {
                      shift-right: [w1213] -> w1202
                      shift-left: w1203 -> [w1213]
                      tunnel: w1201 -> [w1204]
                      stop <- w1208 stop-if-true
                      n162 = local read "Actual output Amplitude (V)"() -> (w1214:dbl)
                      n163 = local read "stop"() -> (w1205:bool)
                      n164 = local read "Abort Change"() -> (w1206:bool)
                      n165 = Subtract(x=w1214, y=w1204) -> (x-y=w1211:dbl)
                      n166 = Absolute Value(x=w1211) -> (abs(x)=w1210:dbl)
                      n167 = Or(x=w1206, y=w1205) -> (x .or. y?=w1207:bool)
                      n168 = Less?(x=w1210, y=0.1) -> (x < y?=w1212:bool)
                      n169 = Or(x=w1212, y=w1207) -> (x .or. y?=w1208:bool)
                    }
                  }
                }
              }
              frame True {
              }
            }
          }
        }
      }
      n170 = local read "# of Steps"() -> (w58:i16[])
      n171 = while {
        stop <- w837 stop-if-true
        # "A.C. added 11/14"
        n172 = Wait (ms)(milliseconds to wait=u32 50) -> ()  [unwired: 1 out]
        n173 = local read "Output waveform"() -> (w834:waveform(dbl))
        n174 = local read "Input waveform"() -> (w835:waveform(dbl))
        n175 = Build Array(w834, w835) -> (→"CONTROLS":waveform(dbl)[])
        n176 = local read "Finished"() -> (w833:bool)
        n177 = local read "Testing"() -> (w828:bool)
        n178 = Or(x=w833, y=w828) -> (x .or. y?=w829:bool)
        n179 = local read "error?"() -> (w836:bool)
        n180 = local read "stop"() -> (w831:bool)
        n181 = And(x=w829, y=w831) -> (x .and. y?=w830:bool)
        n182 = Or(x=w836, y=w830) -> (x .or. y?=w837:bool)
      }
      n183 = call "new counter entry.vi"("error in"=w63) -> ("error out"=w80:errorcluster, "Integer Time"=w79:i64)  [unwired: 9 in]
      n184 = call-poly <vilib>:"DAQmx Create Virtual Channel.vi"("counter"="Det1", "error in"=w63) -> ("task out"=w96:refnum<k21>, "error out"=w89:errorcluster)  [unwired: 12 in]
      n185 = call-poly <vilib>:"DAQmx Create Virtual Channel.vi"("counter"="Det2", "error in"=w63) -> ("task out"=w95:refnum<k21>, "error out"=w90:errorcluster)  [unwired: 12 in]
      n186 = call-poly <vilib>:"DAQmx Create Virtual Channel.vi"("counter"="Det3", "error in"=w63) -> ("task out"=w94:refnum<k21>, "error out"=w93:errorcluster)  [unwired: 12 in]
      n187 = call-poly <vilib>:"DAQmx Create Virtual Channel.vi"("counter"="PSU", "error in"=w63) -> ("task out"=w92:refnum<k21>, "error out"=w91:errorcluster)  [unwired: 12 in]
      n188 = Index Array(array=w58) -> (element #1=w57:i16, element #2=w56:i16, element #3=w48:i16)  [unwired: 3 in]
      n189 = call-poly <vilib>:"DAQmx Create Virtual Channel.vi"("maximum value"=10.0 ("Maximum Value"), "minimum value"=-2.5 ("Minimum Value"), "physical channels"="Physical Input Channels", "error in"=w63) -> ("task out"=w67:refnum<k21>, "error out"=w66:errorcluster)  [unwired: 10 in]
      n190 = call-poly <vilib>:"DAQmx Create Virtual Channel.vi"("maximum value"=10.0 ("Maximum Value"), "minimum value"=0.0 ("Minimum Value"), "physical channels"="Physical Output Channels", "error in"=w63) -> ("task out"=w136:refnum<k21>, "error out"=w135:errorcluster)  [unwired: 10 in]
      n191 = Get Date/Time In Seconds() -> (seconds since 1Jan1904=w78:timestamp)
      n192 = Initialize Array(0.0 ("element"), w57, w56, w48) -> (w59:dbl[][][])
      n193 = call <vilib>:"DAQmx Start Task.vi"("task/channels in"=w96, "error in"=w89) -> ("task out"=w120:refnum<k21>, "error out"=w113:errorcluster)  [unwired: 12 in]
      n194 = call <vilib>:"DAQmx Start Task.vi"("task/channels in"=w95, "error in"=w90) -> ("task out"=w119:refnum<k21>, "error out"=w114:errorcluster)  [unwired: 12 in]
      n195 = call <vilib>:"DAQmx Start Task.vi"("task/channels in"=w94, "error in"=w93) -> ("task out"=w118:refnum<k21>, "error out"=w115:errorcluster)  [unwired: 12 in]
      n196 = call <vilib>:"DAQmx Start Task.vi"("task/channels in"=w92, "error in"=w91) -> ("task out"=w117:refnum<k21>, "error out"=w116:errorcluster)  [unwired: 12 in]
      n197 = To Double Precision Float(number=w78) -> (double precision float=w77:dbl)
      n198 = call-poly <vilib>:"DAQmx Timing.vi"("task/channels in"=w67, "rate"=5000.0, "error in"=w66) -> ("task out"=w72:refnum<k21>, "error out"=w71:errorcluster)  [unwired: 11 in]
      n199 = while {
        shift-right: [w269] -> _
        shift-left: w79 -> [w271]
        shift-right: [w261] -> _
        shift-left: w77 -> [w256]
        shift-right: [w260] -> _
        shift-left: w46 -> [w267]
        shift-right: [w259] -> _
        shift-left: w46 -> [w266]
        shift-right: [w258] -> _
        shift-left: w46 -> [w265]
        shift-right: [w238] -> _
        shift-left: w49 -> [w234]
        shift-right: [w237] -> _
        shift-left: w49 -> [w233]
        shift-right: [w239] -> _
        shift-left: w59 -> [w240]
        shift-right: [w236] -> _
        shift-left: w47 -> [w232]
        shift-right: [w235] -> _
        shift-left: w47 -> [w231]
        shift-right: [w228] -> _
        shift-left: w47 -> [w227]
        shift-right: [w221] -> _
        shift-left: TRUE -> [w222]
        shift-right: [w291] -> w112
        shift-left: w120 -> [w279]
        shift-right: [w281] -> w111
        shift-left: w113 -> [w278]
        shift-right: [w290] -> w110
        shift-left: w119 -> [w277]
        shift-right: [w287] -> w109
        shift-left: w114 -> [w276]
        shift-right: [w289] -> w108
        shift-left: w118 -> [w275]
        shift-right: [w286] -> w107
        shift-left: w115 -> [w274]
        shift-right: [w288] -> w106
        shift-left: w117 -> [w273]
        shift-right: [w285] -> w105
        shift-left: w116 -> [w272]
        shift-right: [w280] -> w87
        shift-left: w80 -> [w270]
        shift-right: [w202] -> _
        shift-left: w49 -> [w201]
        shift-right: [w197] -> _
        shift-left: w47 -> [w210]
        i -> [w212]
        stop <- w282 stop-if-true
        w178 = T8 {"Minimum"=0.0, "Maximum"=0.0, "Increment"=0.0, "Minor Increment"=0.0, "Start"=0.0} ("Scale.Range")
        w179 = T9 {"Minimum"=0.0, "Maximum"=0.0, "Increment"=0.0} ("Data Entry Limits")
        w284 = u32 100  # millisecond multiple
        n200 = local read "stop"() -> (w255:bool)
        n201 = local read "On/Off"() -> (w211:bool)
        n202 = Not(x=w255) -> (.not. x?=w254:bool)
        n203 = Quotient & Remainder(x=w212, y="Cycles to Avg.") -> (x-y*floor(x/y)=w257:i32)  [unwired: 1 out]
        n204 = And(x=w254, y=w211) -> (x .and. y?=w251:bool)
        n205 = Equal To 0?(x=w257) -> (x = 0?=w252:bool)
        n206 = And(x=w252, y=w251) -> (x .and. y?=w253:bool)
        n207 = event shown="[0] Timeout" {
          selector: _ -> [_ _]
          dyn-events: _ -> [_ _]
          timeout: 0 -> [_ _]
          tunnel: [w398 w457] -> w291
          tunnel: [w393 w455] -> w290
          tunnel: [w392 w453] -> w289
          tunnel: [w391 w451] -> w288
          tunnel: [w390 w454] -> w287
          tunnel: [w389 w452] -> w286
          tunnel: [w388 w450] -> w285
          tunnel: [w379 w456] -> w281
          tunnel: [w378 w442] -> w280
          tunnel: w279 -> [w375 w446]
          tunnel: w278 -> [w374 w461]
          tunnel: w277 -> [w373 w447]
          tunnel: w276 -> [w372 w460]
          tunnel: w275 -> [w371 w448]
          tunnel: w274 -> [w370 w459]
          tunnel: w273 -> [w369 w449]
          tunnel: w272 -> [w368 w458]
          tunnel: w271 -> [w358 w445]
          tunnel: w270 -> [w357 w443]
          tunnel: [w355 w444] -> w269
          tunnel: [w351 w441] -> w264
          tunnel: [w350 w441] -> w263
          tunnel: [w349 w441] -> w262
          event Timeout {
            # "Counter Loop"
            n208 = event-data() -> ()  [unwired: 1 in, 2 out]
            n209 = case shown="True" "Reset Counters" {
              tunnel: w375 -> [w413 w440]
              tunnel: [w413 w438] -> w367
              tunnel: w374 -> [w412 w437]
              tunnel: [w412 w435] -> w366
              tunnel: w373 -> [w411 w434]
              tunnel: [w411 w432] -> w365
              tunnel: w372 -> [w410 w431]
              tunnel: [w410 w429] -> w364
              tunnel: w371 -> [w409 w428]
              tunnel: [w409 w426] -> w363
              tunnel: w370 -> [w408 w425]
              tunnel: [w408 w423] -> w362
              tunnel: w369 -> [w407 w422]
              tunnel: [w407 w420] -> w361
              tunnel: w368 -> [w406 w419]
              tunnel: [w406 w417] -> w360
              tunnel: w357 -> [w405 w415]
              tunnel: [w404 w416] -> w355
              tunnel: [w405 w414] -> w356
              tunnel: w358 -> [w404 _]
              frame False {
              }
              frame True {
                n210 = call <vilib>:"DAQmx Stop Task.vi"("task/channels in"=w428, "error in"=w425) -> ("task out"=w427:refnum<k21>, "error out"=w424:errorcluster)  [unwired: 12 in]
                n211 = call <vilib>:"DAQmx Stop Task.vi"("task/channels in"=w434, "error in"=w431) -> ("task out"=w433:refnum<k21>, "error out"=w430:errorcluster)  [unwired: 12 in]
                n212 = call <vilib>:"DAQmx Stop Task.vi"("task/channels in"=w422, "error in"=w419) -> ("task out"=w421:refnum<k21>, "error out"=w418:errorcluster)  [unwired: 12 in]
                n213 = call <vilib>:"DAQmx Stop Task.vi"("task/channels in"=w440, "error in"=w437) -> ("task out"=w439:refnum<k21>, "error out"=w436:errorcluster)  [unwired: 12 in]
                n214 = call "new counter entry.vi"("error in"=w415) -> ("error out"=w414:errorcluster, "Integer Time"=w416:i64)  [unwired: 9 in]
                n215 = call <vilib>:"DAQmx Start Task.vi"("task/channels in"=w421, "error in"=w418) -> ("task out"=w420:refnum<k21>, "error out"=w417:errorcluster)  [unwired: 12 in]
                n216 = call <vilib>:"DAQmx Start Task.vi"("task/channels in"=w427, "error in"=w424) -> ("task out"=w426:refnum<k21>, "error out"=w423:errorcluster)  [unwired: 12 in]
                n217 = call <vilib>:"DAQmx Start Task.vi"("task/channels in"=w433, "error in"=w430) -> ("task out"=w432:refnum<k21>, "error out"=w429:errorcluster)  [unwired: 12 in]
                n218 = call <vilib>:"DAQmx Start Task.vi"("task/channels in"=w439, "error in"=w436) -> ("task out"=w438:refnum<k21>, "error out"=w435:errorcluster)  [unwired: 12 in]
              }
            }
            n219 = call-poly <vilib>:"DAQmx Read.vi"("task/channels in"=w363, "timeout"=10.0, "error in"=w362) -> ("task out"=w392:refnum<k21>, "data"=w349:u32, "error out"=w385:errorcluster)  [unwired: 10 in]
            "Det3" <- w349
            n220 = call-poly <vilib>:"DAQmx Read.vi"("task/channels in"=w367, "timeout"=10.0, "error in"=w366) -> ("task out"=w398:refnum<k21>, "data"=w351:u32, "error out"=w387:errorcluster)  [unwired: 10 in]
            "Det1" <- w351
            n221 = call-poly <vilib>:"DAQmx Read.vi"("task/channels in"=w361, "timeout"=10.0, "error in"=w360) -> ("task out"=w391:refnum<k21>, "data"=w350:u32, "error out"=w384:errorcluster)  [unwired: 10 in]
            "PSU" <- w350
            n222 = call-poly <vilib>:"DAQmx Read.vi"("task/channels in"=w365, "timeout"=10.0, "error in"=w364) -> ("task out"=w393:refnum<k21>, "data"=w376:u32, "error out"=w386:errorcluster)  [unwired: 10 in]
            "Det2" <- w376
            n223 = Divide(x=w376, y=w351) -> (x/y=→"Det2/Det1":dbl)
            n224 = Divide(x=w349, y=w350) -> (x/y=→"PSU/Det3":dbl)
            n225 = Divide(x=w349, y=w351) -> (x/y=→"Det3/Det1":dbl)
            n226 = Bundle("data"=w351, "data"=w376, "data"=w350, "data"=w349) -> (w348:T10)  [unwired: 1 in]
            n227 = Divide(x=w350, y=w376) -> (x/y=→"PSU/Det2":dbl)
            n228 = Cluster To Array(cluster=w348) -> (array=w347:u32[])
            n229 = Not Equal To 0?(x=w347) -> (x != 0?=w346:bool[])
            n230 = Or Array Elements(Boolean array=w346) -> (logical OR=w345:bool)
            n231 = case shown="True" w345 {
              tunnel: [w399 w400] -> w377
              tunnel: w356 -> [w399 w401]
              tunnel: w355 -> [_ w402]
              tunnel: w348 -> [_ w403]
              frame False {
              }
              frame True {
                n232 = call-poly "update counter entry.vi"("error in"=w401, "Integer Time"=w402, "input cluster"=w403) -> ("error out"=w400:errorcluster)  [unwired: 8 in]
              }
            }
            n233 = call <vilib>:"Clear Errors.vi"("error in (no error)"=w387) -> ("error out"=w379:errorcluster)  [unwired: 5 in, 1 out]
            n234 = call <vilib>:"Clear Errors.vi"("error in (no error)"=w386) -> ("error out"=w390:errorcluster)  [unwired: 5 in, 1 out]
            n235 = call <vilib>:"Clear Errors.vi"("error in (no error)"=w385) -> ("error out"=w389:errorcluster)  [unwired: 5 in, 1 out]
            n236 = call <vilib>:"Clear Errors.vi"("error in (no error)"=w384) -> ("error out"=w388:errorcluster)  [unwired: 5 in, 1 out]
            n237 = call "counter_sum.vi"("error in"=w377) -> ("error IO"=w378:errorcluster, "Number of Hours"=→"Hours Run":dbl, "Third Detector Sum"=w354:i64, "First Detector Sum"=w353:i64)  [unwired: 7 in]
            "First detector since\nlast source change:" <- w353
            "Third detector since\nlast source change:" <- w354
            n238 = Divide(x=w354, y=w353) -> (x/y=→"Source Efficiency":dbl)
          }
          event "Counters On/Off": Value Change {
            w441 = u32 0 ("data")
            n239 = event-data() -> ("NewVal"=w462:bool)  [unwired: 1 in, 4 out]
            n240 = case shown="True" w462 {
              tunnel: w461 -> [w482 w494]
              tunnel: w460 -> [w480 w493]
              tunnel: w459 -> [w478 w492]
              tunnel: w458 -> [w476 w491]
              tunnel: [w468 w502] -> w457
              tunnel: [w469 w501] -> w456
              tunnel: [w470 w500] -> w455
              tunnel: [w471 w499] -> w454
              tunnel: [w472 w498] -> w453
              tunnel: [w473 w497] -> w452
              tunnel: [w475 w496] -> w451
              tunnel: [w474 w495] -> w450
              tunnel: w449 -> [w477 w490]
              tunnel: w448 -> [w479 w489]
              tunnel: w447 -> [w481 w488]
              tunnel: w446 -> [w483 w487]
              tunnel: w445 -> [_ w486]
              tunnel: [w467 w486] -> w444
              tunnel: w443 -> [w466 w485]
              tunnel: [w465 w485] -> w442
              frame False {
                n241 = call <vilib>:"DAQmx Stop Task.vi"("task/channels in"=w479, "error in"=w478) -> ("task out"=w472:refnum<k21>, "error out"=w473:errorcluster)  [unwired: 12 in]
                n242 = call <vilib>:"DAQmx Stop Task.vi"("task/channels in"=w481, "error in"=w480) -> ("task out"=w470:refnum<k21>, "error out"=w471:errorcluster)  [unwired: 12 in]
                n243 = call <vilib>:"DAQmx Stop Task.vi"("task/channels in"=w477, "error in"=w476) -> ("task out"=w475:refnum<k21>, "error out"=w474:errorcluster)  [unwired: 12 in]
                n244 = call <vilib>:"DAQmx Stop Task.vi"("task/channels in"=w483, "error in"=w482) -> ("task out"=w468:refnum<k21>, "error out"=w469:errorcluster)  [unwired: 12 in]
                n245 = call "new counter entry.vi"("error in"=w466) -> ("error out"=w465:errorcluster, "Integer Time"=w467:i64)  [unwired: 9 in]
                n246 = property on="Calibrate XY" class="Bool (strict)"("Value"=FALSE ("Calibrate XY"), "DisabledEnum"=T6."Disabled and Grayed Out" ("Disabled")) -> ()  [unwired: 2 in, 2 out]
              }
              frame True {
                n247 = call <vilib>:"DAQmx Start Task.vi"("task/channels in"=w487, "error in"=w494) -> ("task out"=w502:refnum<k21>, "error out"=w501:errorcluster)  [unwired: 12 in]
                n248 = call <vilib>:"DAQmx Start Task.vi"("task/channels in"=w488, "error in"=w493) -> ("task out"=w500:refnum<k21>, "error out"=w499:errorcluster)  [unwired: 12 in]
                n249 = call <vilib>:"DAQmx Start Task.vi"("task/channels in"=w489, "error in"=w492) -> ("task out"=w498:refnum<k21>, "error out"=w497:errorcluster)  [unwired: 12 in]
                n250 = call <vilib>:"DAQmx Start Task.vi"("task/channels in"=w490, "error in"=w491) -> ("task out"=w496:refnum<k21>, "error out"=w495:errorcluster)  [unwired: 12 in]
                n251 = property on="Calibrate XY" class="Bool (strict)"("DisabledEnum"=T6."Enabled" ("Disabled")) -> ()  [unwired: 2 in, 2 out]
              }
            }
          }
        }
        n252 = case shown="True" w253 {
          tunnel: w256 -> [w619 w675]
          tunnel: w267 -> [w610 w674]
          tunnel: w266 -> [w618 w673]
          tunnel: w265 -> [w617 w672]
          tunnel: w264 -> [_ w666]
          tunnel: w263 -> [_ w665]
          tunnel: w262 -> [_ w664]
          tunnel: [w619 w667] -> w261
          tunnel: [w610 w666] -> w260
          tunnel: [w618 w665] -> w259
          tunnel: [w617 w664] -> w258
          tunnel: w240 -> [w614 w659]
          tunnel: w234 -> [_ w647]
          tunnel: w233 -> [_ w646]
          tunnel: w232 -> [w616 w660]
          tunnel: w231 -> [w615 w641]
          tunnel: [w614 w658] -> w220
          tunnel: [w616 w657] -> w230
          tunnel: [w615 w656] -> w229
          tunnel: w227 -> [w613 w653]
          tunnel: [w613 w654] -> w225
          tunnel: w210 -> [w612 w644]
          tunnel: w201 -> [_ w648]
          tunnel: [w612 w645] -> w196
          frame False {
            n253 = local read "Tab Control"() -> (w611:T3)
            n254 = case shown="\"EXY Scan Data\"" w611 {
              frame "Controls", Default {
              }
              frame "EXY Scan Data" {
                w622 = u8 0 ("Z Scale.Scale Fit")
                n255 = local read "Einzel Slice"() -> (w632:dbl)
                n256 = local read "Einzel Vs"() -> (w635:dbl[])
                n257 = local read "Y Slice"() -> (w630:dbl)
                n258 = local read "X Vs"() -> (w634:dbl[])
                n259 = local read "Y Vs"() -> (w633:dbl[])
                n260 = local read "X Slice"() -> (w631:dbl)
                n261 = local read "Rate Data"() -> (w626:dbl[][][])
                n262 = Search 1D Array(1D array=w633, element=w630) -> (index of element=w629:i32)  [unwired: 1 in]
                n263 = Search 1D Array(1D array=w634, element=w631) -> (index of element=w628:i32)  [unwired: 1 in]
                n264 = Search 1D Array(1D array=w635, element=w632) -> (index of element=w627:i32)  [unwired: 1 in]
                n265 = Index Array(array=w626, index (dim 0)=w627) -> (element=w625:dbl[][])  [unwired: 2 in]
                n266 = Array Max & Min(array=w626) -> (max value=w621:dbl, min value=w620:dbl)  [unwired: 2 out]
                n267 = Index Array(array=w626, index (dim 1)=w628) -> (element=w624:dbl[][])  [unwired: 2 in]
                n268 = Index Array(array=w626, index (dim 2)=w629) -> (element=w623:dbl[][])  [unwired: 2 in]
                n269 = local write "Einzel Slice Data"(w625) -> ()
                n270 = local write "Y Slice Data"(w623) -> ()
                n271 = local write "X Slice Data"(w624) -> ()
                n272 = property on="X Slice Data" class="IntGraph (strict)"("ZScale.Maximum"=w621, "ZScale.Minimum"=w620, "ZScale.ScaleFit"=w622) -> ()  [unwired: 2 in, 2 out]
                n273 = property on="Y Slice Data" class="IntGraph (strict)"("ZScale.Maximum"=w621, "ZScale.Minimum"=w620, "ZScale.ScaleFit"=w622) -> ()  [unwired: 2 in, 2 out]
                n274 = property on="Einzel Slice Data" class="IntGraph (strict)"("ZScale.Maximum"=w621, "ZScale.Minimum"=w620, "ZScale.ScaleFit"=w622) -> ()  [unwired: 2 in, 2 out]
              }
            }
          }
          frame True {
            n275 = local read "# of Steps"() -> (w655:i16[])
            n276 = Get Date/Time In Seconds() -> (seconds since 1Jan1904=w676:timestamp)
            n277 = To Double Precision Float(number=w676) -> (double precision float=w667:dbl)
            n278 = Index Array(array=w655, index #1=1 ("index"), index #2=2 ("index")) -> (element #1=w638:i16, element #2=w637:i16)
            n279 = local read "Num Steps"() -> (w651:i16)
            n280 = Subtract(x=w667, y=w675) -> (x-y=w668:dbl)
            n281 = Subtract(x=w666, y=w674) -> (x-y=w671:u32)
            n282 = Decrement(x=w638) -> (x-1=w636:i16)
            n283 = Subtract(x=w665, y=w673) -> (x-y=w670:u32)
            n284 = Decrement(x=w651) -> (x-1=w650:i16)
            n285 = Less?(x=w644, y=w637) -> (x < y?=w643:bool)
            n286 = Equal?(x=w636, y=w641) -> (x = y?=w642:bool)
            n287 = Subtract(x=w664, y=w672) -> (x-y=w669:u32)
            n288 = Less?(x=w653, y=w650) -> (x < y?=w652:bool)
            n289 = Divide(x=w671, y=w668) -> (x/y=→"Det1 Rate":dbl)
            n290 = Divide(x=w670, y=w668) -> (x/y=→"PSU Rate":dbl)
            n291 = Divide(x=w669, y=w668) -> (x/y=w649:dbl)
            "Det3 Rate" <- w649
            n292 = local read "Calibrate XY"() -> (w661:bool)
            n293 = case shown="True" w661 {
              tunnel: w647 -> [_ w702]
              tunnel: w646 -> [_ w701]
              tunnel: w660 -> [w681 w724]
              tunnel: w641 -> [w680 w723]
              tunnel: w659 -> [w682 w722]
              tunnel: [w682 w713] -> w658
              tunnel: w649 -> [_ w721]
              tunnel: [w681 w720] -> w657
              tunnel: [w680 w719] -> w656
              tunnel: w653 -> [w679 w718]
              tunnel: [w679 w717] -> w654
              tunnel: w652 -> [_ w716]
              tunnel: w644 -> [w678 w715]
              tunnel: w648 -> [_ w709]
              tunnel: [w678 w703] -> w645
              tunnel: w643 -> [_ w700]
              tunnel: w642 -> [_ w699]
              frame False {
                n294 = local read "Tab Control"() -> (w677:T3)
                n295 = case shown="\"EXY Scan Data\"" w677 {
                  frame "Controls", Default {
                  }
                  frame "EXY Scan Data" {
                    w686 = u8 0 ("Z Scale.Scale Fit")
                    n296 = local read "Einzel Slice"() -> (w697:dbl)
                    n297 = local read "Einzel Vs"() -> (w698:dbl[])
                    n298 = local read "X Slice"() -> (w695:dbl)
                    n299 = local read "Y Slice"() -> (w693:dbl)
                    n300 = local read "X Vs"() -> (w696:dbl[])
                    n301 = local read "Y Vs"() -> (w694:dbl[])
                    n302 = Search 1D Array(1D array=w694, element=w693) -> (index of element=w690:i32)  [unwired: 1 in]
                    n303 = Search 1D Array(1D array=w696, element=w695) -> (index of element=w691:i32)  [unwired: 1 in]
                    n304 = Search 1D Array(1D array=w698, element=w697) -> (index of element=w692:i32)  [unwired: 1 in]
                    n305 = local read "Rate Data"() -> (w685:dbl[][][])
                    n306 = Index Array(array=w685, index (dim 0)=w692) -> (element=w689:dbl[][])  [unwired: 2 in]
                    n307 = Array Max & Min(array=w685) -> (max value=w684:dbl, min value=w683:dbl)  [unwired: 2 out]
                    n308 = Index Array(array=w685, index (dim 1)=w691) -> (element=w688:dbl[][])  [unwired: 2 in]
                    n309 = Index Array(array=w685, index (dim 2)=w690) -> (element=w687:dbl[][])  [unwired: 2 in]
                    n310 = local write "Einzel Slice Data"(w689) -> ()
                    n311 = local write "X Slice Data"(w688) -> ()
                    n312 = local write "Y Slice Data"(w687) -> ()
                    n313 = property on="Einzel Slice Data" class="IntGraph (strict)"("ZScale.Maximum"=w684, "ZScale.Minimum"=w683, "ZScale.ScaleFit"=w686) -> ()  [unwired: 2 in, 2 out]
                    n314 = property on="Y Slice Data" class="IntGraph (strict)"("ZScale.Maximum"=w684, "ZScale.Minimum"=w683, "ZScale.ScaleFit"=w686) -> ()  [unwired: 2 in, 2 out]
                    n315 = property on="X Slice Data" class="IntGraph (strict)"("ZScale.Maximum"=w684, "ZScale.Minimum"=w683, "ZScale.ScaleFit"=w686) -> ()  [unwired: 2 in, 2 out]
                  }
                }
              }
              frame True {
                n316 = case shown="True" w700 {
                  tunnel: w724 -> [w727 w776]
                  tunnel: w723 -> [w726 w761]
                  tunnel: w722 -> [w744 w775]
                  tunnel: w721 -> [w743 w759]
                  tunnel: [w727 w774] -> w720
                  tunnel: [w726 w773] -> w719
                  tunnel: w718 -> [w742 w763]
                  tunnel: [w741 w758] -> w717
                  tunnel: w716 -> [_ w772]
                  tunnel: w702 -> [w740 w771]
                  tunnel: w701 -> [w739 w770]
                  tunnel: w715 -> [w730 w769]
                  tunnel: [w738 w768] -> w713
                  tunnel: w709 -> [w737 w767]
                  tunnel: [w729 w766] -> w703
                  tunnel: w699 -> [_ w762]
                  frame True {
                    w732 = T5 4 items=["Get", "Set X", "Set Y", "Set XY", "Internal"] ("Ring")
                    n317 = Index Array(array=w737, index=w727) -> (element=w731:dbl)
                    n318 = Index Array(array=w740, index=w726) -> (element=w735:dbl)
                    n319 = Decrement(x=w730) -> (x-1=w728:i32)
                    n320 = Index Array(array=w739, index=w730) -> (element=w736:dbl)
                    n321 = property on="Einzel Voltage" class="DigNum (strict)"("Val(Sgnl)"=w731) -> ()  [unwired: 2 in, 2 out]
                    n322 = Less Than 0?(x=w728) -> (x < 0?=w725:bool)
                    n323 = call "XYVoltage.vi"("X Voltage"=w735, "Y Voltage"=w736, "Ring"=w732) -> ("X Voltage 2"=w734:dbl, "Y Voltage 2"=w733:dbl)  [unwired: 5 in, 1 out]
                    n324 = property on="Y Voltage" class="DigNum (strict)"("Val(Sgnl)"=w733) -> ()  [unwired: 2 in, 2 out]
                    n325 = property on="X Voltage" class="DigNum (strict)"("Val(Sgnl)"=w734) -> ()  [unwired: 2 in, 2 out]
                    n326 = case shown="False" w725 {
                      tunnel: w744 -> [w754 w756]
                      tunnel: [w753 w756] -> w738
                      tunnel: w728 -> [w750 _]
                      tunnel: w726 -> [w751 _]
                      tunnel: w743 -> [w747 _]
                      tunnel: w742 -> [w749 w755]
                      tunnel: [w746 w755] -> w741
                      tunnel: w727 -> [w752 _]
                      frame False {
                        n327 = local read "Cal Test?"() -> (w745:bool)
                        n328 = Increment(x=w749) -> (x+1=w746:i32)
                        n329 = Select(t=w746, s=w745, f=w747) -> (s? t:f=w748:dbl)
                        n330 = Replace Array Subset(array=w754, new element=w748, index (dim 0)=w752, index (dim 1)=w751, index (dim 2)=w750) -> (w753:dbl[][][])
                      }
                      frame True {
                      }
                    }
                    n331 = Increment(x=w730) -> (x+1=w729:i32)
                  }
                  frame False {
                    n332 = Decrement(x=w769) -> (x-1=w764:i32)
                    n333 = Increment(x=w763) -> (x+1=w758:i32)
                    n334 = Select(t=w758, s="Cal Test?", f=w759) -> (s? t:f=w760:dbl)
                    n335 = Replace Array Subset(array=w775, new element=w760, index (dim 0)=w776, index (dim 1)=w761, index (dim 2)=w764) -> (w765:dbl[][][])
                    n336 = case shown="True" w772 {
                      tunnel: w771 -> [w781 w827]
                      tunnel: w770 -> [w780 w826]
                      tunnel: w776 -> [_ w810]
                      tunnel: w761 -> [_ w818]
                      tunnel: [w778 w815] -> w773
                      tunnel: w765 -> [w779 w820]
                      tunnel: [w779 w820] -> w768
                      tunnel: [w778 w812] -> w774
                      tunnel: w767 -> [w777 w819]
                      tunnel: w769 -> [_ _]
                      tunnel: [w778 w808] -> w766
                      tunnel: w762 -> [_ w811]
                      frame False {
                        w778 = 0
                        n337 = Less Or Equal To 0?(x=w779) -> (x <= 0?=w783:bool[][][])
                        n338 = And Array Elements(Boolean array=w783) -> (logical AND=w782:bool)
                        n339 = case shown="False" w782 {
                          tunnel: w779 -> [w801 _]
                          tunnel: w781 -> [w797 _]
                          tunnel: w780 -> [w796 _]
                          tunnel: w777 -> [w786 _]
                          frame False {
                            w793 = T5 4 items=["Get", "Set X", "Set Y", "Set XY", "Internal"] ("Ring")
                            n340 = Array Max & Min(array=w801) -> (max index (indices)=w800:i32[])  [unwired: 3 out]
                            n341 = Index Array(array=w800, index #1=0 ("index"), index #2=1 ("index"), index #3=2 ("index")) -> (element #1=w787:i32, element #2=w788:i32, element #3=w789:i32)
                            n342 = Index Array(array=w796, index=w789) -> (element=w795:dbl)
                            n343 = Index Array(array=w786, index=w787) -> (element=w785:dbl)
                            n344 = Index Array(array=w797, index=w788) -> (element=w794:dbl)
                            n345 = property on="Einzel Voltage" class="DigNum (strict)"("Val(Sgnl)"=w785) -> ()  [unwired: 2 in, 2 out]
                            n346 = call "XYVoltage.vi"("X Voltage"=w794, "Y Voltage"=w795, "Ring"=w793) -> ("X Voltage 2"=w792:dbl, "Y Voltage 2"=w791:dbl)  [unwired: 5 in, 1 out]
                            n347 = property on="X Voltage" class="DigNum (strict)"("Val(Sgnl)"=w792) -> ()  [unwired: 2 in, 2 out]
                            n348 = property on="Y Voltage" class="DigNum (strict)"("Val(Sgnl)"=w791) -> ()  [unwired: 2 in, 2 out]
                          }
                          frame True {
                            w805 = T5 4 items=["Get", "Set X", "Set Y", "Set XY", "Internal"] ("Ring")
                            n349 = local read "Old Einzel"() -> (w802:dbl)
                            n350 = call "XYVoltage.vi"("X Voltage"=0.0, "Y Voltage"=0.0, "Ring"=w805) -> ("X Voltage 2"=w804:dbl, "Y Voltage 2"=w803:dbl)  [unwired: 5 in, 1 out]
                            n351 = property on="X Voltage" class="DigNum (strict)"("Val(Sgnl)"=w804) -> ()  [unwired: 2 in, 2 out]
                            n352 = property on="Y Voltage" class="DigNum (strict)"("Val(Sgnl)"=w803) -> ()  [unwired: 2 in, 2 out]
                            n353 = property on="Einzel Voltage" class="DigNum (strict)"("Val(Sgnl)"=w802) -> ()  [unwired: 2 in, 2 out]
                          }
                        }
                        n354 = local write "Calibrate XY"(FALSE ("Calibrate XY")) -> ()
                      }
                      frame True {
                        w816 = 0
                        w821 = T5 4 items=["Get", "Set X", "Set Y", "Set XY", "Internal"] ("Ring")
                        n355 = Increment(x=w818) -> (x+1=w814:i32)
                        n356 = Increment(x=w810) -> (x+1=w809:i32)
                        n357 = Select(t=w809, s=w811, f=w810) -> (s? t:f=w812:i32)
                        n358 = Select(t=0, s=w811, f=w814) -> (s? t:f=w815:i32)
                        n359 = Index Array(array=w827, index=w815) -> (element=w824:dbl)
                        n360 = Index Array(array=w819, index=w812) -> (element=w817:dbl)
                        n361 = Increment(x=w816) -> (x+1=w808:i32)
                        n362 = Index Array(array=w826, index=w816) -> (element=w825:dbl)
                        n363 = call "XYVoltage.vi"("X Voltage"=w824, "Y Voltage"=w825, "Ring"=w821) -> ("X Voltage 2"=w822:dbl, "Y Voltage 2"=w823:dbl)  [unwired: 5 in, 1 out]
                        n364 = property on="Y Voltage" class="DigNum (strict)"("Val(Sgnl)"=w823) -> ()  [unwired: 2 in, 2 out]
                        n365 = property on="X Voltage" class="DigNum (strict)"("Val(Sgnl)"=w822) -> ()  [unwired: 2 in, 2 out]
                        n366 = property on="Einzel Voltage" class="DigNum (strict)"("Val(Sgnl)"=w817) -> ()  [unwired: 2 in, 2 out]
                      }
                    }
                  }
                }
                "Rate Data" <- w713
                n367 = Search 1D Array(1D array=w702, element="X Slice") -> (index of element=w704:i32)  [unwired: 1 in]
                n368 = Search 1D Array(1D array=w701, element="Y Slice") -> (index of element=w705:i32)  [unwired: 1 in]
                n369 = Search 1D Array(1D array=w709, element="Einzel Slice") -> (index of element=w708:i32)  [unwired: 1 in]
                n370 = Index Array(array=w713, index (dim 0)=w708) -> (element=→"Einzel Slice Data":dbl[][])  [unwired: 2 in]
                n371 = Index Array(array=w713, index (dim 2)=w705) -> (element=→"Y Slice Data":dbl[][])  [unwired: 2 in]
                n372 = Index Array(array=w713, index (dim 1)=w704) -> (element=→"X Slice Data":dbl[][])  [unwired: 2 in]
              }
            }
          }
        }
        n373 = Unbundle By Name("Things to Scan") -> ("Einzel"=w171:bool, "X"=w170:bool, "Y"=w169:bool)
        n374 = case shown="False" w171 {
          tunnel: [w330 w342] -> w175
          tunnel: "Calibrate XY" -> [_ w339]
          frame False {
            w327 = 10.0 ("y")
            n375 = local read "Einzel Voltage"() -> (w337:dbl)
            n376 = local read "# of Steps"() -> (w334:i16[])
            n377 = Increment(x=w337) -> (x+1=w328:dbl)
            n378 = Less Or Equal?(x=w328, y=w327) -> (x <= y?=w329:bool)
            n379 = Select(t=w328, s=w329, f=w327) -> (s? t:f=w326:dbl)
            n380 = Replace Array Subset(array=w334, new element=i16 1 ("new element/subarray"), index=0) -> (w333:i16[])
            n381 = Build Array(w337, w326) -> (w336:dbl[])
            n382 = local write "# of Steps"(w333) -> ()
            n383 = property on="Ein. Range" class="Arr (strict)"("DisabledEnum"=2 ("element"), "Value"=w336) -> (error out=w330:errorcluster)  [unwired: 2 in, 1 out]
          }
          frame True {
            n384 = Select(t=2, s=w339, f=0 ("element")) -> (s? t:f=w340:i32)
            n385 = property on="Ein. Range" class="Arr (strict)"("DisabledEnum"=w340) -> (error out=w342:errorcluster)  [unwired: 2 in, 1 out]
          }
        }
        n386 = case shown="False" w170 {
          tunnel: [w313 w325] -> w176
          tunnel: "Calibrate XY" -> [_ w322]
          frame False {
            w311 = 2.5 ("y")
            n387 = local read "# of Steps"() -> (w317:i16[])
            n388 = local read "X Voltage"() -> (w320:dbl)
            n389 = Increment(x=w320) -> (x+1=w310:dbl)
            n390 = Less Or Equal?(x=w310, y=w311) -> (x <= y?=w312:bool)
            n391 = Select(t=w310, s=w312, f=w311) -> (s? t:f=w309:dbl)
            n392 = Replace Array Subset(array=w317, new element=i16 1 ("new element/subarray"), index=1) -> (w316:i16[])
            n393 = Build Array(w320, w309) -> (w319:dbl[])
            n394 = local write "# of Steps"(w316) -> ()
            n395 = property on="X Range" class="Arr (strict)"("DisabledEnum"=2 ("element"), "Value"=w319) -> (error out=w313:errorcluster)  [unwired: 2 in, 1 out]
          }
          frame True {
            n396 = Select(t=2, s=w322, f=0 ("element")) -> (s? t:f=w323:i32)
            n397 = property on="X Range" class="Arr (strict)"("DisabledEnum"=w323) -> (error out=w325:errorcluster)  [unwired: 2 in, 1 out]
          }
        }
        n398 = case shown="False" w169 {
          tunnel: [w296 w308] -> w177
          tunnel: "Calibrate XY" -> [_ w306]
          frame False {
            w294 = 2.5 ("y")
            n399 = local read "# of Steps"() -> (w300:i16[])
            n400 = local read "Y Voltage"() -> (w302:dbl)
            n401 = Increment(x=w302) -> (x+1=w293:dbl)
            n402 = Less Or Equal?(x=w293, y=w294) -> (x <= y?=w295:bool)
            n403 = Select(t=w293, s=w295, f=w294) -> (s? t:f=w292:dbl)
            n404 = Replace Array Subset(array=w300, new element=i16 1 ("new element/subarray"), index=2) -> (w299:i16[])
            n405 = Build Array(w302, w292) -> (w303:dbl[])
            n406 = local write "# of Steps"(w299) -> ()
            n407 = property on="Y Range" class="Arr (strict)"("DisabledEnum"=2 ("element"), "Value"=w303) -> (error out=w296:errorcluster)  [unwired: 2 in, 1 out]
          }
          frame True {
            n408 = Select(t=2, s=w306, f=0 ("element")) -> (s? t:f=w307:i32)
            n409 = property on="Y Range" class="Arr (strict)"("DisabledEnum"=w307) -> (error out=w308:errorcluster)  [unwired: 2 in, 1 out]
          }
        }
        n410 = call-poly <userlib>:"Data Changed__ogtk.vi"("Boolean"="Calibrate XY") -> ("Changed"=w185:bool)
        n411 = And(x=w185, y="Calibrate XY") -> (x .and. y?=w186:bool)
        n412 = Index Array(array="# of Steps") -> (element #1=w153:i16, element #2=w155:i16, element #3=w158:i16)  [unwired: 3 in]
        n413 = Multiply Array Elements(1:"# of Steps") -> (0:w226:i16)
        "Num Steps" <- w226
        n414 = case shown="True" w186 {
          frame False {
          }
          frame True {
            n415 = local read "Einzel Voltage"() -> (→"Old Einzel":dbl)
          }
        }
        n416 = Subtract(x=w226, y=w225) -> (x-y=→"Steps to go":i32)
        n417 = Merge Errors(w175, w176, w177) -> (w174:errorcluster)
        n418 = Decrement(x=w153) -> (x-1=w183:i16)
        n419 = Index Array(array="Ein. Range") -> (element #1=w209:dbl, element #2=w208:dbl)  [unwired: 2 in]
        n420 = Index Array(array="X Range") -> (element #1=w249:dbl, element #2=w250:dbl)  [unwired: 2 in]
        n421 = Decrement(x=w155) -> (x-1=w215:i16)
        n422 = Index Array(array="Y Range") -> (element #1=w248:dbl, element #2=w247:dbl)  [unwired: 2 in]
        n423 = Subtract(x=w209, y=w208) -> (x-y=w207:dbl)
        n424 = Decrement(x=w158) -> (x-1=w217:i16)
        n425 = Equal To 0?(x=w183) -> (x = 0?=w182:bool)
        n426 = Subtract(x=w249, y=w250) -> (x-y=w245:dbl)
        n427 = Subtract(x=w248, y=w247) -> (x-y=w246:dbl)
        n428 = Equal To 0?(x=w215) -> (x = 0?=w181:bool)
        n429 = Array Max & Min(array="Y Range") -> (max value=w192:dbl, min value=w191:dbl)  [unwired: 2 out]
        n430 = Array Max & Min(array="X Range") -> (max value=w190:dbl, min value=w189:dbl)  [unwired: 2 out]
        n431 = Equal To 0?(x=w217) -> (x = 0?=w180:bool)
        n432 = Select(t=i16 1, s=w182, f=w183) -> (s? t:f=w205:i16)
        n433 = Select(t=i16 1, s=w181, f=w215) -> (s? t:f=w213:i16)
        n434 = Array Max & Min(array="Ein. Range") -> (max value=w195:dbl, min value=w194:dbl)  [unwired: 2 out]
        n435 = Divide(x=w245, y=w213) -> (x/y=w244:dbl)
        n436 = Divide(x=w207, y=w205) -> (x/y=w204:dbl)
        n437 = Select(t=i16 1, s=w180, f=w217) -> (s? t:f=w216:i16)
        n438 = Absolute Value(x=w244) -> (abs(x)=w164:dbl)
        n439 = Absolute Value(x=w204) -> (abs(x)=w167:dbl)
        n440 = Divide(x=w246, y=w216) -> (x/y=w243:dbl)
        n441 = Absolute Value(x=w243) -> (abs(x)=w160:dbl)
        n442 = Equal To 0?(x=w167) -> (x = 0?=w152:bool)
        n443 = Equal To 0?(x=w164) -> (x = 0?=w156:bool)
        n444 = Equal To 0?(x=w160) -> (x = 0?=w159:bool)
        n445 = Select(t=0.1, s=w152, f=w167) -> (s? t:f=w166:dbl)
        n446 = Select(t=0.1, s=w156, f=w164) -> (s? t:f=w163:dbl)
        n447 = Select(t=i16 1, s=w152, f=w153) -> (s? t:f=w150:i16)
        n448 = Select(t=i16 1, s=w156, f=w155) -> (s? t:f=w149:i16)
        n449 = Select(t=0.1, s=w159, f=w160) -> (s? t:f=w161:dbl)
        n450 = Bundle(cluster=w178, "Minimum"=w189, "Maximum"=w190, "Increment"=w163, "Minor Increment"=w163, "Start"=w189) -> (w188:T8)
        n451 = Bundle(cluster=w179, "Minimum"=w189, "Maximum"=w190, "Increment"=w163) -> (w200:T9)
        n452 = Select(t=i16 1, s=w159, f=w158) -> (s? t:f=w148:i16)
        n453 = Bundle(cluster=w179, "Minimum"=w191, "Maximum"=w192, "Increment"=w161) -> (w199:T9)
        n454 = Bundle(cluster=w178, "Minimum"=w191, "Maximum"=w192, "Increment"=w161, "Minor Increment"=w161, "Start"=w191) -> (w187:T8)
        n455 = Bundle(cluster=w179, "Minimum"=w194, "Maximum"=w195, "Increment"=w166) -> (w198:T9)
        n456 = Bundle(cluster=w178, "Minimum"=w194, "Maximum"=w195, "Increment"=w166, "Minor Increment"=w166, "Start"=w194) -> (w193:T8)
        n457 = Build Array(w150, w149, w148) -> (w147:i16[])
        n458 = case shown="True" "Calibrate XY" {
          tunnel: w148 -> [w505 w572]
          tunnel: w191 -> [_ w563]
          tunnel: w189 -> [_ w558]
          tunnel: w163 -> [_ w568]
          tunnel: w161 -> [_ w562]
          tunnel: [w507 w560] -> w238
          tunnel: [w507 w561] -> w237
          tunnel: [w509 w576] -> w239
          tunnel: [w508 w575] -> w236
          tunnel: [w508 w574] -> w235
          tunnel: w220 -> [_ w576]
          tunnel: w230 -> [_ w575]
          tunnel: w229 -> [_ w574]
          tunnel: w149 -> [w504 w573]
          tunnel: [w508 w571] -> w228
          tunnel: w225 -> [_ w571]
          tunnel: w222 -> [_ w557]
          tunnel: [TRUE FALSE] -> w221
          tunnel: w194 -> [_ w564]
          tunnel: w166 -> [_ w567]
          tunnel: w150 -> [w506 w566]
          tunnel: [w507 w565] -> w202
          tunnel: w200 -> [_ w554]
          tunnel: w199 -> [_ w553]
          tunnel: w198 -> [_ w555]
          tunnel: w196 -> [_ w559]
          tunnel: [w508 w559] -> w197
          tunnel: w193 -> [_ w530]
          tunnel: w188 -> [_ w522]
          tunnel: w187 -> [_ w514]
          tunnel: w182 -> [_ w539]
          tunnel: w181 -> [_ w538]
          tunnel: w180 -> [_ w537]
          tunnel: w174 -> [_ _]
          frame False {
            w503 = T6."Enabled" ("Disabled")
            w508 = 0
            w507 = dbl[] []
            n459 = property on="# of Steps" class="Arr (strict)"("DisabledEnum"=w503) -> ()  [unwired: 2 in, 2 out]
            n460 = property on="X Voltage" class="DigNum (strict)"("DisabledEnum"=w503) -> ()  [unwired: 2 in, 2 out]
            n461 = property on="Y Voltage" class="DigNum (strict)"("DisabledEnum"=w503) -> ()  [unwired: 2 in, 2 out]
            n462 = property on="Things to Scan" class="Clust (strict)"("DisabledEnum"=w503) -> ()  [unwired: 2 in, 2 out]
            n463 = property on="Einzel Voltage" class="DigNum (strict)"("DisabledEnum"=w503) -> ()  [unwired: 2 in, 2 out]
            n464 = Initialize Array(0.0 ("element"), w506, w504, w505) -> (w509:dbl[][][])
          }
          frame True {
            w540 = u8 1 ("Z Scale.Scale Fit")
            w512 = T6."Disabled and Grayed Out" ("Disabled")
            n465 = for {
              N: w573 -> [_]
              tunnel: w568 -> [w608]
              tunnel: w558 -> [w606]
              tunnel: [w605] -> w560 mode=indexing
              i -> [w609]
              n466 = Multiply(x=w608, y=w609) -> (x*y=w607:dbl)
              n467 = Add(x=w606, y=w607) -> (x+y=w605:dbl)
            }
            "X Vs" <- w560
            n468 = for {
              N: w566 -> [_]
              tunnel: w567 -> [w595]
              tunnel: w564 -> [w594]
              tunnel: [w592] -> w565 mode=indexing
              i -> [w596]
              n469 = Multiply(x=w595, y=w596) -> (x*y=w593:dbl)
              n470 = Add(x=w594, y=w593) -> (x+y=w592:dbl)
            }
            "Einzel Vs" <- w565
            n471 = for {
              N: w572 -> [_]
              tunnel: w562 -> [w603]
              tunnel: w563 -> [w602]
              tunnel: [w600] -> w561 mode=indexing
              i -> [w604]
              n472 = Multiply(x=w603, y=w604) -> (x*y=w601:dbl)
              n473 = Add(x=w602, y=w601) -> (x+y=w600:dbl)
            }
            "Y Vs" <- w561
            n474 = Equal To 0?(x=w571) -> (x = 0?=w556:bool)
            n475 = And(x=w556, y=w557) -> (x .and. y?=w570:bool)
            n476 = case shown="True" w570 {
              tunnel: w558 -> [_ w599]
              tunnel: w563 -> [_ w598]
              tunnel: w564 -> [_ w597]
              frame False {
              }
              frame True {
                n477 = property on="X Voltage" class="DigNum (strict)"("Val(Sgnl)"=w599) -> ()  [unwired: 2 in, 2 out]
                n478 = property on="Einzel Voltage" class="DigNum (strict)"("Val(Sgnl)"=w597) -> ()  [unwired: 2 in, 2 out]
                n479 = property on="Y Voltage" class="DigNum (strict)"("Val(Sgnl)"=w598) -> ()  [unwired: 2 in, 2 out]
              }
            }
            n480 = property on="Einzel Slice" class="Slide (strict)"("Data Range"=w555, "Scale.Range"=w530) -> ()  [unwired: 2 in, 2 out]
            n481 = property on="X Slice" class="Slide (strict)"("Data Range"=w554, "Scale.Range"=w522) -> ()  [unwired: 2 in, 2 out]
            n482 = property on="Y Slice" class="Slide (strict)"("Data Range"=w553, "Scale.Range"=w514) -> ()  [unwired: 2 in, 2 out]
            n483 = property on="Einzel Voltage" class="DigNum (strict)"("DisabledEnum"=w512) -> ()  [unwired: 2 in, 2 out]
            n484 = property on="Ein. Range" class="Arr (strict)"("DisabledEnum"=w512) -> ()  [unwired: 2 in, 2 out]
            n485 = property on="X Range" class="Arr (strict)"("DisabledEnum"=w512) -> ()  [unwired: 2 in, 2 out]
            n486 = Unbundle(w555) -> ("Minimum"=w552:dbl, "Increment"=w551:dbl)  [unwired: 1 out]
            n487 = Unbundle(w553) -> ("Minimum"=w548:dbl, "Increment"=w547:dbl)  [unwired: 1 out]
            n488 = Unbundle(w554) -> ("Minimum"=w550:dbl, "Increment"=w549:dbl)  [unwired: 1 out]
            n489 = Bundle("Minimum"=w552, "Increment"=w551) -> (w546:cluster{"Minimum":dbl, "Increment":dbl})  [unwired: 1 in]
            n490 = Bundle("Minimum"=w550, "Increment"=w549) -> (w545:cluster{"Minimum":dbl, "Increment":dbl})  [unwired: 1 in]
            n491 = Bundle("Minimum"=w548, "Increment"=w547) -> (w544:cluster{"Minimum":dbl, "Increment":dbl})  [unwired: 1 in]
            n492 = property on="Y Range" class="Arr (strict)"("DisabledEnum"=w512) -> ()  [unwired: 2 in, 2 out]
            n493 = property on="Y Voltage" class="DigNum (strict)"("DisabledEnum"=w512) -> ()  [unwired: 2 in, 2 out]
            n494 = Unbundle(w514) -> ("Minimum"=w520:dbl, "Maximum"=w519:dbl, "Increment"=w517:dbl, "Minor Increment"=w516:dbl, "Start"=w515:dbl)
            n495 = Unbundle(w530) -> ("Minimum"=w536:dbl, "Maximum"=w535:dbl, "Increment"=w533:dbl, "Minor Increment"=w532:dbl, "Start"=w531:dbl)
            n496 = Unbundle(w522) -> ("Minimum"=w528:dbl, "Maximum"=w527:dbl, "Increment"=w525:dbl, "Minor Increment"=w524:dbl, "Start"=w523:dbl)
            n497 = property on="# of Steps" class="Arr (strict)"("DisabledEnum"=w512) -> ()  [unwired: 2 in, 2 out]
            n498 = property on="X Voltage" class="DigNum (strict)"("DisabledEnum"=w512) -> ()  [unwired: 2 in, 2 out]
            n499 = Add(x=w519, y=w517) -> (x+y=w518:dbl)
            n500 = Add(x=w535, y=w533) -> (x+y=w534:dbl)
            n501 = Add(x=w527, y=w525) -> (x+y=w526:dbl)
            n502 = Bundle("Minimum"=w520, w518, "Increment"=w517, "Minor Increment"=w516, "Start"=w515) -> (w513:T11)  [unwired: 1 in]
            n503 = Bundle("Minimum"=w536, w534, "Increment"=w533, "Minor Increment"=w532, "Start"=w531) -> (w529:T11)  [unwired: 1 in]
            n504 = Bundle("Minimum"=w528, w526, "Increment"=w525, "Minor Increment"=w524, "Start"=w523) -> (w521:T11)  [unwired: 1 in]
            n505 = property on="Things to Scan" class="Clust (strict)"("DisabledEnum"=w512) -> ()  [unwired: 2 in, 2 out]
            n506 = case shown="False" w539 {
              tunnel: w529 -> [w587 w589]
              tunnel: [w587 w589] -> w543
              frame False {
                n507 = property on="Einzel Slice" class="Slide (strict)"("DisabledEnum"=0) -> ()  [unwired: 2 in, 2 out]
              }
              frame True {
                n508 = Unbundle By Name(w589) -> ("Minimum"=w590:dbl)
                n509 = property on="Einzel Slice" class="Slide (strict)"("DisabledEnum"=2, "Value"=w590) -> ()  [unwired: 2 in, 2 out]
              }
            }
            n510 = case shown="False" w538 {
              tunnel: w521 -> [w582 w585]
              tunnel: [w582 w585] -> w542
              frame False {
                n511 = property on="X Slice" class="Slide (strict)"("DisabledEnum"=0) -> ()  [unwired: 2 in, 2 out]
              }
              frame True {
                n512 = Unbundle By Name(w585) -> ("Minimum"=w584:dbl)
                n513 = property on="X Slice" class="Slide (strict)"("DisabledEnum"=2, "Value"=w584) -> ()  [unwired: 2 in, 2 out]
              }
            }
            n514 = case shown="False" w537 {
              tunnel: w513 -> [w577 w580]
              tunnel: [w577 w580] -> w541
              frame False {
                n515 = property on="Y Slice" class="Slide (strict)"("DisabledEnum"=0) -> ()  [unwired: 2 in, 2 out]
              }
              frame True {
                n516 = Unbundle By Name(w580) -> ("Minimum"=w579:dbl)
                n517 = property on="Y Slice" class="Slide (strict)"("DisabledEnum"=2, "Value"=w579) -> ()  [unwired: 2 in, 2 out]
              }
            }
            n518 = property on="Y Slice Data" class="IntGraph (strict)"("XScale.Ofst&Mult"=w546, "XScale.Range"=w543, "YScale.Ofst&Mult"=w545, "YScale.Range"=w542, "ZScale.ScaleFit"=w540) -> ()  [unwired: 2 in, 2 out]
            n519 = property on="X Slice Data" class="IntGraph (strict)"("XScale.Ofst&Mult"=w546, "XScale.Range"=w543, "YScale.Ofst&Mult"=w544, "YScale.Range"=w541, "ZScale.ScaleFit"=w540) -> ()  [unwired: 2 in, 2 out]
            n520 = property on="Einzel Slice Data" class="IntGraph (strict)"("XScale.Ofst&Mult"=w545, "XScale.Range"=w542, "YScale.Ofst&Mult"=w544, "YScale.Range"=w541, "ZScale.ScaleFit"=w540) -> ()  [unwired: 2 in, 2 out]
          }
        }
        n521 = local write "# of Steps"(w147) -> ()
        n522 = Wait Until Next ms Multiple(millisecond multiple=w284) -> ()  [unwired: 1 out]
        n523 = local read "stop"() -> (w218:bool)
        n524 = local read "error?"() -> (w283:bool)
        n525 = Or(x=w218, y=w283) -> (x .or. y?=w282:bool)
      }
      n526 = property class="DAQmx Write"(reference=w136, error in=w135, "Regeneration Mode"=w137) -> (reference out=w134:refnum<k21>, error out=w133:errorcluster)
      n527 = property class="DAQmx Read"(reference=w72, error in=w71, "ReadAllAvailSamp"=w74, "AutoStart"=w74, "OverWrite"=w73) -> (reference out=w64:refnum<k21>, error out=w62:errorcluster)
      n528 = while {
        shift-right: [w857] -> w61
        shift-left: w64 -> [w858]
        shift-right: [w842] -> w76
        shift-left: w62 -> [w855]
        stop <- w856 stop-if-true
        w862 = 2
        # "If rate exceeds threshold, play alarm sound."
        # "Monitoring Loop"
        n529 = local read "stop"() -> (w852:bool)
        n530 = local read "Finished"() -> (w877:bool)
        n531 = call <vilib>:"DAQmx Start Task.vi"("task/channels in"=w858, "error in"=w855) -> ("task out"=w863:refnum<k21>, "error out"=w864:errorcluster)  [unwired: 12 in]
        n532 = local read "Testing"() -> (w854:bool)
        n533 = And(x=w852, y=w877) -> (x .and. y?=w876:bool)
        n534 = call-poly <vilib>:"DAQmx Read.vi"("task/channels in"=w863, "number of samples per channel"=1000, "error in"=w864) -> ("task out"=w865:refnum<k21>, "data"=w860:waveform(dbl)[], "error out"=w866:errorcluster)  [unwired: 10 in]
        n535 = local read "error?"() -> (w861:bool)
        n536 = And(x=w854, y=w852) -> (x .and. y?=w853:bool)
        n537 = call <vilib>:"DAQmx Stop Task.vi"("task/channels in"=w865, "error in"=w866) -> ("task out"=w857:refnum<k21>, "error out"=w875:errorcluster)  [unwired: 12 in]
        n538 = Index Array(array=w860) -> (element #1=w851:waveform(dbl), element #2=w850:waveform(dbl), element #3=w849:waveform(dbl), element #4=w848:waveform(dbl), element #5=w847:waveform(dbl), element #6=w846:waveform(dbl))  [unwired: 6 in]
        "Input waveform" <- w851
        n539 = Or(x=w861, y=w876) -> (x .or. y?=w859:bool)
        n540 = Or(x=w853, y=w859) -> (x .or. y?=w856:bool)
        n541 = call-poly <vilib>:"Mean.vi"("X"=w846) -> ("mean"=→"Current":dbl)  [unwired: 1 out]
        n542 = Multiply(x=w849, y=w862) -> (x*y=w871:waveform(dbl))
        n543 = Multiply(x=w850, y=w862) -> (x*y=w869:waveform(dbl))
        n544 = call-poly <vilib>:"Mean.vi"("X"=w847) -> ("mean"=→"Actual Steerer X (kV)":dbl)  [unwired: 1 out]
        n545 = call-poly <vilib>:"Mean.vi"("X"=w848) -> ("mean"=→"Actual Steerer Y (kV)":dbl)  [unwired: 1 out]
        n546 = call-poly <vilib>:"Amplitude and Levels.vi"("error in (no error)"=w875, "signal in"=w851) -> ("error out"=w839:errorcluster, "amplitude"=→"Tube Drive":dbl)  [unwired: 6 in, 2 out]
        n547 = call-poly <vilib>:"Mean.vi"("X"=w871) -> ("mean"=→"Actual Needle (kV)":dbl)  [unwired: 1 out]
        n548 = call-poly <vilib>:"Mean.vi"("X"=w869) -> ("mean"=→"Actual Einzel (kV)":dbl)  [unwired: 1 out]
        n549 = property on="Det1 Rate" class="DigNum (strict)"() -> ("Value"=w844:dbl)  [unwired: 2 in, 2 out]
        n550 = Greater?(x=w844, y="Alarm Threshold") -> (0:w840:bool)
        n551 = case shown="True" w840 {
          tunnel: [w878 w881] -> w841
          tunnel: w839 -> [w878 w879]
          frame False {
          }
          frame True {
            # "3 is the code for alarm"
            n552 = call "Play_Sound.vi"("error in (no error)"=w879, "Sound Type"=3) -> ("error out"=w881:errorcluster)
          }
        }
        n553 = Merge Errors(w839, w841) -> (w842:errorcluster)
      }
      n554 = call-poly <vilib>:"DAQmx Timing.vi"("task/channels in"=w134, "sample mode"=w146, "rate"=250000.0 ("Sample Clock Rate"), "error in"=w133) -> ("task out"=w140:refnum<k21>, "error out"=w125:errorcluster)  [unwired: 10 in]
      n555 = property class="DAQmx Timing"(reference=w140, error in=w125) -> (reference out=w128:refnum<k21>, error out=w88:errorcluster, "Sample Clock:Rate"=w132:dbl)
      "Actual Sample Clock Rate" <- w132
      n556 = Get Date/Time In Seconds() -> (seconds since 1Jan1904=w53:timestamp)
      n557 = Bundle By Name(cluster=cluster{"Fs":dbl, "#s":dbl} {"Fs"=1000.0, "#s"=1000.0} ("sampling info"), "#s"=w44, "Fs"=w132) -> (w138:cluster{"Fs":dbl, "#s":dbl})
      n558 = call "LV_to_int_time.vi"("Time Stamp"=w53) -> ("Integer Time"=w52:i64)  [unwired: 8 in, 1 out]
      n559 = while {
        tunnel: w138 -> [w1293]
        tunnel: w132 -> [w1291]
        tunnel: w44 -> [w1278]
        shift-right: [w1290] -> w131
        shift-left: w128 -> [w1288]
        shift-right: [w1286] -> w127
        shift-left: w88 -> [w1295]
        shift-right: [w1240] -> _
        shift-left: w54 -> [w1247]
        shift-right: [w1239] -> _
        shift-left: w54 -> [w1246]
        shift-right: [w1238] -> _
        shift-left: w54 -> [w1245]
        shift-right: [w1237] -> _
        shift-left: w54 -> [w1244]
        shift-right: [w1236] -> _
        shift-left: w54 -> [w1243]
        shift-right: [w1235] -> _
        shift-left: w54 -> [w1242]
        shift-right: [w1234] -> _
        shift-left: w54 -> [w1241]
        shift-right: [w1230] -> _
        shift-left: w52 -> [w1231]
        i -> [w1294]
        stop <- w1287 stop-if-true
        w1272 = 0.0 ("t")
        w1280 = T2 {"Integer Timestamp"=0, "Einzel Voltage"=0.05, "Needle Voltage"=1.0, "Frequency"=0.0, "Width (ms) : 0.1 "=0.0, "Desired Amplitude (V)"=0.0, "X Voltage"=0.0, "Y Voltage"=0.0, "Settings ID"="", "ID#"=0}  # Dust Source Controls
        w1281 = 1
        w1285 = T7 0 items=["no dialog", "OK message", "continue or stop message", "OK message + warnings", "continue/stop + warnings"] ("type of dialog (OK msg:1)")
        w1284 = FALSE ("Blinking")
        # "On criteria - 0: Needle Voltage, 1: Desired Amplitude, 2: Width, 3: Frequency"
        # "Event structure to ramp up or ramp down (depending on what you want) pelletron controls"
        # "Throttling stuff"
        # "Output loop"
        n560 = property on="Actual Needle Output (V)" class="DigNum (strict)"("Blinking"=w1284) -> ()  [unwired: 2 in, 2 out]
        n561 = property on="Actual Y Output (V)" class="DigNum (strict)"("Blinking"=w1284) -> ()  [unwired: 2 in, 2 out]
        n562 = property on="Actual X Output (V)" class="DigNum (strict)"("Blinking"=w1284) -> ()  [unwired: 2 in, 2 out]
        n563 = property on="Actual output Amplitude (V)" class="DigNum (strict)"("Blinking"=w1284) -> ()  [unwired: 2 in, 2 out]
        n564 = property on="Actual Einzel Output (V)" class="DigNum (strict)"("Blinking"=w1284) -> ()  [unwired: 2 in, 2 out]
        n565 = Reciprocal(x=w1291) -> (1/x=w1292:dbl)
        n566 = global read "throttle.vi" "Throttle"() -> (w1248:bool)
        n567 = call-poly <userlib>:"Data Changed__ogtk.vi"("Boolean"=w1248) -> ("Changed"=w1250:bool)
        n568 = case shown="False" w1250 {
          tunnel: w1248 -> [_ w1297]
          tunnel: "Frequency" -> [_ w1296]
          frame False {
          }
          frame True {
            n569 = case shown="True" w1297 {
              tunnel: w1296 -> [_ w1298]
              frame False {
              }
              frame True {
                "Freq. Before Throttle" <- w1298
              }
            }
          }
        }
        n570 = event shown="[1] \"X Voltage\", \"Y Voltage\": Value Change" {
          selector: _ -> [_ _]
          dyn-events: _ -> [_ _]
          timeout: 1 -> [_ _]
          tunnel: [w1322 w1323] -> w1271
          event Timeout {
            w1322 = T5 0 items=["Get", "Set X", "Set Y", "Set XY", "Internal"] ("Ring")
            n571 = event-data() -> ()  [unwired: 1 in, 2 out]
          }
          event "X Voltage", "Y Voltage": Value Change {
            w1323 = T5 4 items=["Get", "Set X", "Set Y", "Set XY", "Internal"] ("Ring")
            n572 = event-data() -> ()  [unwired: 1 in, 2 out]
          }
        }
        n573 = global read "throttle from query.vi" "Throttle Q"() -> (w1273:bool)
        n574 = Or(x=w1273, y=w1248) -> (x .or. y?=w1274:bool)
        n575 = Divide(x="Einzel Voltage", y=w1281) -> (x/y=w1282:dbl)
        n576 = call "XYVoltage.vi"("X Voltage"="X Voltage", "Y Voltage"="Y Voltage", "Ring"=w1271) -> ("X Voltage 2"=w1219:dbl, "Y Voltage 2"=w1217:dbl, "Ring 2"=w1269:T5)  [unwired: 5 in]
        n577 = Bundle("Einzel Voltage"="Einzel Voltage", "X Voltage"="X Voltage", "Y Voltage"="Y Voltage") -> (→"Einzel and Steering":T1)  [unwired: 1 in]
        n578 = case shown="1" w1269 {
          tunnel: w1219 -> [_ w1328 w1332 w1335 _]
          tunnel: w1217 -> [_ w1327 w1330 w1333 _]
          tunnel: [FALSE TRUE TRUE TRUE FALSE] -> w1268
          frame 0, Default {
          }
          frame 1 {
            w1325 = T5 4 items=["Get", "Set X", "Set Y", "Set XY", "Internal"] ("Ring")
            n579 = property on="X Voltage" class="DigNum (strict)"("Val(Sgnl)"=w1328) -> ()  [unwired: 2 in, 2 out]
            n580 = call "XYVoltage.vi"("X Voltage"=w1328, "Y Voltage"=w1327, "Ring"=w1325) -> ()  [unwired: 5 in, 3 out]
          }
          frame 2 {
            w1329 = T5 4 items=["Get", "Set X", "Set Y", "Set XY", "Internal"] ("Ring")
            n581 = property on="Y Voltage" class="DigNum (strict)"("Val(Sgnl)"=w1330) -> ()  [unwired: 2 in, 2 out]
            n582 = call "XYVoltage.vi"("X Voltage"=w1332, "Y Voltage"=w1330, "Ring"=w1329) -> ()  [unwired: 5 in, 3 out]
          }
          frame 3 {
            w1334 = T5 2 items=["Get", "Set X", "Set Y", "Set XY", "Internal"] ("Ring")
            n583 = property on="X Voltage" class="DigNum (strict)"("Val(Sgnl)"=w1335) -> ()  [unwired: 2 in, 2 out]
            n584 = property on="Y Voltage" class="DigNum (strict)"("Value"=w1333) -> ()  [unwired: 2 in, 2 out]
            n585 = call "XYVoltage.vi"("X Voltage"=w1335, "Y Voltage"=w1333, "Ring"=w1334) -> ()  [unwired: 5 in, 3 out]
          }
          frame 4 {
          }
        }
        n586 = local read "Freq. Before Throttle"() -> (w1251:dbl)
        n587 = Implies(1:w1248, 2:w1250) -> (0:w1249:bool)
        n588 = Select(t=T6."Disabled and Grayed Out" ("Disabled"), s=w1274, f=T6."Enabled" ("Disabled")) -> (s? t:f=w1275:T6)
        n589 = property on="Frequency" class="DigNum (strict)"("DisabledEnum"=w1275) -> ()  [unwired: 2 in, 2 out]
        n590 = Select(t=w1272, s=w1273, f="Frequency") -> (s? t:f=w1266:dbl)
        n591 = Select(t=w1272, s=w1248, f=w1266) -> (s? t:f=w1262:dbl)
        n592 = Select(t=w1262, s=w1249, f=w1251) -> (s? t:f=w1252:dbl)
        n593 = Divide(x="Needle Voltage", y=w1281) -> (x/y=w1283:dbl)
        n594 = call "scale xy steering.vi"("-2.5 to 2.5 V input"=w1219) -> ("0 to 9 V output"=w1218:dbl)  [unwired: 1 in, 1 out]
        n595 = call "scale xy steering.vi"("-2.5 to 2.5 V input"=w1217) -> ("0 to 9 V output"=w1216:dbl)  [unwired: 1 in, 1 out]
        n596 = call-poly <userlib>:"Data Changed__ogtk.vi"("DBL"=w1252) -> ("Changed"=w1267:bool)
        n597 = case shown="True" w1267 {
          tunnel: w1252 -> [_ w1321]
          frame False {
          }
          frame True {
            n598 = property on="Frequency" class="DigNum (strict)"("Val(Sgnl)"=w1321) -> ()  [unwired: 2 in, 2 out]
          }
        }
        n599 = Bundle By Name(cluster=w1280, "Desired Amplitude (V)"="Desired Amplitude (V)", "Width (ms) : 0.1"="Width (ms) : 0.1", "Frequency"=w1252, "Einzel Voltage"="Einzel Voltage", "X Voltage"=w1219, "Y Voltage"=w1217, "Needle Voltage"="Needle Voltage") -> (→"output cluster":T2)
        n600 = Build Array("Needle Voltage", "Desired Amplitude (V)", "Width (ms) : 0.1", w1252) -> (w1261:dbl[])
        n601 = Greater?(x=w1261, y=dbl[] [1.0, 0.0, 0.0, 0.0]) -> (0:w1259:bool[])
        n602 = And Array Elements(Boolean array=w1259) -> (logical AND=w1232:bool)
        "On/Off" <- w1232
        n603 = event shown="[3] \"Y Voltage\": Value Change" {
          selector: _ -> [_ _ _ _ _ _ _ _ _]
          dyn-events: _ -> [_ _ _ _ _ _ _ _ _]
          timeout: 100 -> [_ _ _ _ _ _ _ _ _]
          tunnel: w1293 -> [w1351 w1413 w1540 w1662 w1781 w1869 w1990 w2103 w2218]
          tunnel: w1295 -> [w1375 w1405 w1555 w1677 w1776 w1868 w1966 w2079 w2194]
          tunnel: w1252 -> [w1346 w1428 w1556 w1678 w1799 w1847 w1946 w2105 w2176]
          tunnel: "Width (ms) : 0.1" -> [w1347 w1429 w1557 w1679 w1800 w1846 w1948 w2060 w2220]
          tunnel: [w1374 w1403 w1558 w1680 w1775 w1859 w1964 w2077 w2192] -> w1258
          tunnel: w1288 -> [w1373 w1427 w1554 w1676 w1798 w1863 w1991 w2104 w2219]
          tunnel: "Desired Amplitude (V)" -> [w1349 w1402 w1529 w1651 w1773 w1853 w1947 w2061 w2175]
          tunnel: w1278 -> [w1355 w1417 w1545 w1667 w1789 w1865 w1978 w2091 w2206]
          tunnel: w1292 -> [w1354 w1416 w1544 w1666 w1788 w1866 w1977 w2090 w2205]
          tunnel: w1282 -> [w1366 w1385 w1551 w1673 w1795 w1848 w1987 w2100 w2215]
          tunnel: [w1365 w1426 w1553 w1675 w1797 w1864 w1986 w2099 w2214] -> w1290
          tunnel: w1218 -> [w1358 w1423 _ w1669 w1791 _ w1984 w2097 w2212]
          tunnel: w1216 -> [w1359 w1420 w1547 _ w1785 _ w1982 w2095 w2210]
          tunnel: [FALSE ("y") FALSE ("y") FALSE ("y") FALSE ("y") FALSE ("y") TRUE ("y") FALSE ("y") FALSE ("y") FALSE ("y")] -> w1255
          tunnel: w1283 -> [w1353 w1415 w1542 w1664 _ w1852 w1974 w2087 w2202]
          tunnel: w1268 -> [_ _ w1530 w1652 _ _ _ _ _]
          tunnel: w1247 -> [w1345 w1396 w1528 w1649 w1771 _ w1962 w2075 w2190]
          tunnel: w1246 -> [w1344 w1395 w1526 w1648 w1772 _ w1961 w2074 w2189]
          tunnel: w1245 -> [w1343 w1401 w1525 w1647 w1770 _ w1963 w2073 w2188]
          tunnel: w1244 -> [w1342 w1400 w1524 w1646 w1769 _ w1960 w2072 w2191]
          tunnel: w1243 -> [w1341 w1399 w1523 w1645 w1768 _ w1959 w2076 w2187]
          tunnel: w1242 -> [w1340 w1398 w1527 w1644 w1767 _ w1958 w2071 w2186]
          tunnel: w1241 -> [w1339 w1397 w1522 w1650 w1766 _ w1957 w2070 w2185]
          tunnel: [w1345 w1387 w1528 w1649 w1771 w1854 w1962 w2075 w2190] -> w1240
          tunnel: [w1344 w1395 w1526 w1648 w1760 w1854 w1961 w2074 w2189] -> w1239
          tunnel: [w1343 w1401 w1525 w1647 w1770 w1854 w1951 w2073 w2188] -> w1238
          tunnel: [w1342 w1400 w1524 w1646 w1769 w1854 w1960 w2072 w2179] -> w1237
          tunnel: [w1341 w1399 w1523 w1645 w1768 w1854 w1959 w2062 w2187] -> w1236
          tunnel: [w1340 w1398 w1516 w1644 w1767 w1854 w1958 w2071 w2186] -> w1235
          tunnel: [w1339 w1397 w1522 w1638 w1766 w1854 w1957 w2070 w2185] -> w1234
          event Timeout {
            w1348 = FALSE ("Blinking")
            n604 = event-data() -> ()  [unwired: 1 in, 2 out]
            n605 = local write "Actual X Output (V)"(w1358) -> ()
            n606 = local write "Actual Y Output (V)"(w1359) -> ()
            n607 = local write "Actual Needle Output (V)"(w1353) -> ()
            n608 = local write "Actual Einzel Output (V)"(w1366) -> ()
            n609 = local write "Actual output Amplitude (V)"(w1349) -> ()
            n610 = call "Gen_Square_0to10V.vi"("sampling info"=w1351, "error in (no error)"=w1375, "Width (ms)"=w1347, "amplitude"=w1349, "frequency"=w1346) -> ("error out"=w1370:errorcluster, "signal out"=w1350:waveform(dbl))  [unwired: 5 in]
            n611 = Initialize Array(w1358, w1355) -> (w1363:dbl[])
            n612 = Initialize Array(w1359, w1355) -> (w1361:dbl[])
            n613 = Initialize Array(w1353, w1355) -> (w1356:dbl[])
            n614 = Initialize Array(w1366, w1355) -> (w1367:dbl[])
            n615 = local write "Actual output width (ms)"(w1347) -> ()
            n616 = local write "Actual output Frequency"(w1346) -> ()
            n617 = local write "Output waveform"(w1350) -> ()
            n618 = Bundle By Name("Y"=w1363, "dt"=w1354) -> (w1362:waveform(dbl))  [unwired: 1 in]
            n619 = Bundle By Name("Y"=w1361, "dt"=w1354) -> (w1360:waveform(dbl))  [unwired: 1 in]
            n620 = Bundle By Name("Y"=w1356, "dt"=w1354) -> (w1352:waveform(dbl))  [unwired: 1 in]
            n621 = Bundle By Name("Y"=w1367, "dt"=w1354) -> (w1364:waveform(dbl))  [unwired: 1 in]
            n622 = Merge Signals(w1350, w1364, w1362, w1360, w1352) -> (w1368:dynamicdata)
            n623 = local read "Tab Control"() -> (w1338:T3)
            n624 = call-poly <vilib>:"DAQmx Write.vi"("task/channels in"=w1373, "data"=w1368, "error in"=w1370) -> ("task out"=w1372:refnum<k21>, "error out"=w1369:errorcluster)  [unwired: 10 in, 1 out]
            n625 = case shown="\"EXY Scan Data\"" w1338 {
              frame "Controls", Default {
              }
              frame "EXY Scan Data" {
              }
              frame "Status" {
                n626 = Unbundle By Name("Maximums") -> ("Width"=w1377:dbl, "Freq."=w1376:dbl)
                n627 = property on="Frequency" class="DigNum (strict)"("Maximum"=w1376) -> ()  [unwired: 2 in, 2 out]
                n628 = property on="Width (ms) : 0.1" class="DigNum (strict)"("Maximum"=w1377) -> ()  [unwired: 2 in, 2 out]
              }
            }
            n629 = First Call?() -> (First Call?: T/F=w1371:bool)
            n630 = case shown="True" w1371 {
              tunnel: [w1379 w1384] -> w1374
              tunnel: [w1380 w1383] -> w1365
              tunnel: w1372 -> [w1380 w1382]
              tunnel: w1369 -> [w1379 w1381]
              frame False {
              }
              frame True {
                n631 = call <vilib>:"DAQmx Start Task.vi"("task/channels in"=w1382, "error in"=w1381) -> ("task out"=w1383:refnum<k21>, "error out"=w1384:errorcluster)  [unwired: 12 in]
              }
            }
            n632 = property on="Actual output Amplitude (V)" class="DigNum (strict)"("Blinking"=w1348) -> ()  [unwired: 2 in, 2 out]
            n633 = property on="Actual X Output (V)" class="DigNum (strict)"("Blinking"=w1348) -> ()  [unwired: 2 in, 2 out]
            n634 = property on="Actual Needle Output (V)" class="DigNum (strict)"("Blinking"=w1348) -> ()  [unwired: 2 in, 2 out]
            n635 = property on="Actual Einzel Output (V)" class="DigNum (strict)"("Blinking"=w1348) -> ()  [unwired: 2 in, 2 out]
            n636 = property on="Actual Y Output (V)" class="DigNum (strict)"("Blinking"=w1348) -> ()  [unwired: 2 in, 2 out]
            n637 = property on="Actual output width (ms)" class="DigNum (strict)"("Blinking"=w1348) -> ()  [unwired: 2 in, 2 out]
            n638 = property on="Actual output Frequency" class="DigNum (strict)"("Blinking"=w1348) -> ()  [unwired: 2 in, 2 out]
          }
          event "Einzel Voltage": Value Change {
            w1411 = 0.05 ("y")
            n639 = event-data() -> ("NewVal"=w1388:dbl)  [unwired: 1 in, 4 out]
            n640 = local write "Actual X Output (V)"(w1423) -> ()
            n641 = local write "Actual Y Output (V)"(w1420) -> ()
            n642 = local write "Actual Needle Output (V)"(w1415) -> ()
            n643 = Greater?(x=w1388, y=w1396) -> (0:w1412:bool)
            n644 = Subtract(x=w1396, y=w1388) -> (x-y=w1407:dbl)
            n645 = Subtract(x=w1388, y=w1396) -> (x-y=w1409:dbl)
            n646 = Initialize Array(w1423, w1417) -> (w1425:dbl[])
            n647 = Initialize Array(w1420, w1417) -> (w1422:dbl[])
            n648 = Initialize Array(w1415, w1417) -> (w1418:dbl[])
            n649 = Greater?(x=w1407, y=w1409) -> (0:w1410:bool)
            n650 = Bundle By Name("Y"=w1425, "dt"=w1416) -> (w1424:waveform(dbl))  [unwired: 1 in]
            n651 = Bundle By Name("Y"=w1422, "dt"=w1416) -> (w1421:waveform(dbl))  [unwired: 1 in]
            n652 = Bundle By Name("Y"=w1418, "dt"=w1416) -> (w1414:waveform(dbl))  [unwired: 1 in]
            n653 = Select(t=w1407, s=w1410, f=w1409) -> (s? t:f=w1406:dbl)
            n654 = local read "Calibrate XY"() -> (w1386:bool)
            n655 = Divide(x=w1406, y=w1411) -> (x/y=w1408:dbl)
            n656 = To Long Integer(number=w1408) -> (32bit integer=w1389:i32)
            n657 = case shown="False" w1386 {
              tunnel: w1429 -> [w1448 w1512]
              tunnel: w1428 -> [w1447 w1511]
              tunnel: w1427 -> [w1446 w1510]
              tunnel: [w1445 w1509] -> w1426
              tunnel: w1424 -> [w1444 w1508]
              tunnel: w1421 -> [w1443 w1507]
              tunnel: w1417 -> [w1442 w1506]
              tunnel: w1416 -> [w1441 w1505]
              tunnel: w1414 -> [w1440 w1504]
              tunnel: w1413 -> [w1439 w1503]
              tunnel: w1412 -> [w1438 _]
              tunnel: w1411 -> [w1437 _]
              tunnel: w1405 -> [w1436 w1502]
              tunnel: [w1435 w1501] -> w1404
              tunnel: w1402 -> [w1434 w1500]
              tunnel: w1396 -> [w1433 _]
              tunnel: [w1432 w1491] -> w1391
              tunnel: [w1431 w1499] -> w1390
              tunnel: w1389 -> [w1430 _]
              tunnel: w1385 -> [_ w1491]
              frame False {
                n658 = for {
                  N: w1430 -> [_]
                  tunnel: w1437 -> [w1483]
                  tunnel: w1433 -> [w1482]
                  tunnel: w1441 -> [w1481]
                  tunnel: w1442 -> [w1480]
                  tunnel: [w1479] -> w1435
                  tunnel: w1448 -> [w1472]
                  tunnel: w1434 -> [w1460]
                  tunnel: w1447 -> [w1475]
                  tunnel: w1436 -> [w1474]
                  tunnel: w1444 -> [w1470]
                  tunnel: w1443 -> [w1469]
                  tunnel: w1440 -> [w1467]
                  shift-right: [w1478] -> w1445
                  shift-left: w1446 -> [w1473]
                  tunnel: w1439 -> [w1466]
                  tunnel: w1438 -> [w1462]
                  tunnel: [w1457] -> w1432
                  tunnel: [w1455] -> w1431
                  i -> [w1484]
                  stop <- w1455 stop-if-true
                  n659 = local write "Actual output Amplitude (V)"(w1460) -> ()
                  n660 = call "Gen_Square_0to10V.vi"("sampling info"=w1466, "error in (no error)"=w1474, "Width (ms)"=w1472, "amplitude"=w1460, "frequency"=w1475) -> ("error out"=w1476:errorcluster, "signal out"=w1461:waveform(dbl))  [unwired: 5 in]
                  n661 = Increment(x=w1484) -> (x+1=w1485:i32)
                  n662 = property on="Actual Einzel Output (V)" class="DigNum (strict)"("Blinking"=TRUE) -> ()  [unwired: 2 in, 2 out]
                  n663 = local write "Output waveform"(w1461) -> ()
                  n664 = Multiply(x=w1483, y=w1485) -> (x*y=w1464:dbl)
                  n665 = Negate(x=w1464) -> (-x=w1463:dbl)
                  n666 = Select(t=w1464, s=w1462, f=w1463) -> (s? t:f=w1465:dbl)
                  n667 = Add(x=w1482, y=w1465) -> (x+y=w1453:dbl)
                  n668 = Less Than 0?(x=w1453) -> (x < 0?=w1459:bool)
                  n669 = Select(t=0.0, s=w1459, f=w1453) -> (s? t:f=w1457:dbl)
                  n670 = local write "Actual Einzel Output (V)"(w1457) -> ()
                  n671 = Initialize Array(w1457, w1480) -> (w1450:dbl[])
                  n672 = In Range and Coerce(upper limit=10.0, x=w1450, lower limit=0.0) -> (coerced(x)=w1449:dbl[])  [unwired: 1 out]
                  n673 = Bundle By Name("Y"=w1449, "dt"=w1481) -> (w1471:waveform(dbl))  [unwired: 1 in]
                  n674 = local read "Abort Change"() -> (w1456:bool)
                  n675 = local read "stop"() -> (w1454:bool)
                  n676 = Or(x=w1454, y=w1456) -> (x .or. y?=w1455:bool)
                  n677 = Merge Signals(w1461, w1471, w1470, w1469, w1467) -> (w1477:dynamicdata)
                  n678 = case shown="True" w1455 {
                    tunnel: w1457 -> [_ w1486]
                    frame False {
                    }
                    frame True {
                      n679 = local write "Einzel Voltage"(w1486) -> ()
                    }
                  }
                  n680 = call-poly <vilib>:"DAQmx Write.vi"("task/channels in"=w1473, "data"=w1477, "error in"=w1476) -> ("task out"=w1478:refnum<k21>, "error out"=w1479:errorcluster)  [unwired: 10 in, 1 out]
                }
              }
              frame True {
                n681 = local write "Actual output Amplitude (V)"(w1500) -> ()
                n682 = call "Gen_Square_0to10V.vi"("sampling info"=w1503, "error in (no error)"=w1502, "Width (ms)"=w1512, "amplitude"=w1500, "frequency"=w1511) -> ("error out"=w1497:errorcluster, "signal out"=w1494:waveform(dbl))  [unwired: 5 in]
                n683 = property on="Actual Einzel Output (V)" class="DigNum (strict)"("Blinking"=TRUE) -> ()  [unwired: 2 in, 2 out]
                n684 = local write "Output waveform"(w1494) -> ()
                n685 = local write "Actual Einzel Output (V)"(w1491) -> ()
                n686 = Initialize Array(w1491, w1506) -> (w1488:dbl[])
                n687 = In Range and Coerce(upper limit=10.0, x=w1488, lower limit=0.0) -> (coerced(x)=w1487:dbl[])  [unwired: 1 out]
                n688 = Bundle By Name("Y"=w1487, "dt"=w1505) -> (w1496:waveform(dbl))  [unwired: 1 in]
                n689 = local read "Abort Change"() -> (w1493:bool)
                n690 = local read "stop"() -> (w1492:bool)
                n691 = Or(x=w1492, y=w1493) -> (x .or. y?=w1499:bool)
                n692 = Merge Signals(w1494, w1496, w1508, w1507, w1504) -> (w1498:dynamicdata)
                n693 = case shown="True" w1499 {
                  tunnel: w1491 -> [_ w1513]
                  frame False {
                  }
                  frame True {
                    n694 = local write "Einzel Voltage"(w1513) -> ()
                  }
                }
                n695 = call-poly <vilib>:"DAQmx Write.vi"("task/channels in"=w1510, "data"=w1498, "error in"=w1497) -> ("task out"=w1509:refnum<k21>, "error out"=w1501:errorcluster)  [unwired: 10 in, 1 out]
              }
            }
            n696 = Equal To 0?(x=w1389) -> (x = 0?=w1393:bool)
            n697 = Not(x=w1390) -> (.not. x?=w1394:bool)
            n698 = Merge Errors(w1404) -> (w1403:errorcluster)
            n699 = Or(x=w1394, y=w1393) -> (x .or. y?=w1392:bool)
            n700 = Select(t=w1388, s=w1392, f=w1391) -> (s? t:f=w1387:dbl)
          }
          event "X Voltage": Value Change {
            w1537 = 0.05 ("y")
            n701 = event-data() -> ("NewVal"=w1515:dbl)  [unwired: 1 in, 4 out]
            n702 = local write "Actual Y Output (V)"(w1547) -> ()
            n703 = local write "Actual Needle Output (V)"(w1542) -> ()
            n704 = local write "Actual Einzel Output (V)"(w1551) -> ()
            n705 = Greater?(x=w1515, y=w1527) -> (0:w1539:bool)
            n706 = Subtract(x=w1515, y=w1527) -> (x-y=w1533:dbl)
            n707 = Subtract(x=w1527, y=w1515) -> (x-y=w1536:dbl)
            n708 = Initialize Array(w1547, w1545) -> (w1549:dbl[])
            n709 = Initialize Array(w1542, w1545) -> (w1543:dbl[])
            n710 = Initialize Array(w1551, w1545) -> (w1552:dbl[])
            n711 = Greater?(x=w1533, y=w1536) -> (0:w1538:bool)
            n712 = Bundle By Name("Y"=w1549, "dt"=w1544) -> (w1548:waveform(dbl))  [unwired: 1 in]
            n713 = Bundle By Name("Y"=w1543, "dt"=w1544) -> (w1541:waveform(dbl))  [unwired: 1 in]
            n714 = Bundle By Name("Y"=w1552, "dt"=w1544) -> (w1550:waveform(dbl))  [unwired: 1 in]
            n715 = Select(t=w1533, s=w1538, f=w1536) -> (s? t:f=w1534:dbl)
            n716 = Divide(x=w1534, y=w1537) -> (x/y=w1535:dbl)
            n717 = local read "Calibrate XY"() -> (w1532:bool)
            n718 = To Long Integer(number=w1535) -> (32bit integer=w1514:i32)
            n719 = Or(x=w1532, y=w1530) -> (x .or. y?=w1531:bool)
            n720 = case shown="True" w1531 {
              tunnel: [w1577 w1622] -> w1558
              tunnel: w1557 -> [w1576 w1635]
              tunnel: w1529 -> [w1575 w1634]
              tunnel: w1556 -> [w1574 w1633]
              tunnel: w1555 -> [w1573 w1632]
              tunnel: w1554 -> [w1572 w1631]
              tunnel: [w1571 w1623] -> w1553
              tunnel: w1550 -> [w1570 w1630]
              tunnel: w1548 -> [w1569 w1629]
              tunnel: w1545 -> [w1568 w1628]
              tunnel: w1544 -> [w1567 w1627]
              tunnel: w1541 -> [w1566 w1626]
              tunnel: w1540 -> [w1565 w1625]
              tunnel: w1539 -> [w1564 _]
              tunnel: w1537 -> [w1563 _]
              tunnel: w1514 -> [w1562 _]
              tunnel: w1527 -> [w1561 _]
              tunnel: w1515 -> [_ w1615]
              tunnel: [w1560 w1614] -> w1517
              tunnel: [w1559 FALSE ("Abort Change")] -> w1518
              frame False {
                n721 = for {
                  N: w1562 -> [_]
                  tunnel: w1563 -> [w1607]
                  tunnel: w1561 -> [w1606]
                  tunnel: w1567 -> [w1605]
                  tunnel: w1568 -> [w1604]
                  tunnel: [w1603] -> w1577
                  tunnel: w1576 -> [w1585]
                  tunnel: w1575 -> [w1584]
                  tunnel: w1574 -> [w1599]
                  tunnel: w1573 -> [w1598]
                  tunnel: w1570 -> [w1595]
                  tunnel: w1569 -> [w1593]
                  tunnel: w1566 -> [w1592]
                  shift-right: [w1602] -> w1571
                  shift-left: w1572 -> [w1597]
                  tunnel: w1565 -> [w1591]
                  tunnel: w1564 -> [w1587]
                  tunnel: [w1579] -> w1560
                  tunnel: [w1583] -> w1559
                  i -> [w1608]
                  stop <- w1583 stop-if-true
                  n722 = local write "Actual output Amplitude (V)"(w1584) -> ()
                  n723 = call "Gen_Square_0to10V.vi"("sampling info"=w1591, "error in (no error)"=w1598, "Width (ms)"=w1585, "amplitude"=w1584, "frequency"=w1599) -> ("error out"=w1600:errorcluster, "signal out"=w1586:waveform(dbl))  [unwired: 5 in]
                  n724 = Increment(x=w1608) -> (x+1=w1609:i32)
                  n725 = property on="Actual X Output (V)" class="DigNum (strict)"("Blinking"=TRUE) -> ()  [unwired: 2 in, 2 out]
                  n726 = local write "Output waveform"(w1586) -> ()
                  n727 = Multiply(x=w1607, y=w1609) -> (x*y=w1589:dbl)
                  n728 = Negate(x=w1589) -> (-x=w1590:dbl)
                  n729 = Select(t=w1589, s=w1587, f=w1590) -> (s? t:f=w1588:dbl)
                  n730 = Add(x=w1606, y=w1588) -> (x+y=w1579:dbl)
                  n731 = call "scale xy steering.vi"("-2.5 to 2.5 V input"=w1579) -> ("0 to 9 V output"=w1578:dbl)  [unwired: 1 in, 1 out]
                  n732 = local write "Actual X Output (V)"(w1578) -> ()
                  n733 = Initialize Array(w1578, w1604) -> (w1580:dbl[])
                  n734 = Bundle By Name("Y"=w1580, "dt"=w1605) -> (w1594:waveform(dbl))  [unwired: 1 in]
                  n735 = local read "Abort Change"() -> (w1582:bool)
                  n736 = Merge Signals(w1586, w1595, w1594, w1593, w1592) -> (w1601:dynamicdata)
                  n737 = local read "stop"() -> (w1581:bool)
                  n738 = Or(x=w1581, y=w1582) -> (x .or. y?=w1583:bool)
                  n739 = call-poly <vilib>:"DAQmx Write.vi"("task/channels in"=w1597, "data"=w1601, "error in"=w1600) -> ("task out"=w1602:refnum<k21>, "error out"=w1603:errorcluster)  [unwired: 10 in, 1 out]
                  n740 = case shown="True" w1583 {
                    tunnel: w1579 -> [_ w1611]
                    frame False {
                    }
                    frame True {
                      w1610 = T5 4 items=["Get", "Set X", "Set Y", "Set XY", "Internal"] ("Ring")
                      w1613 = T5 0 items=["Get", "Set X", "Set Y", "Set XY", "Internal"] ("Ring")
                      n741 = local write "X Voltage"(w1611) -> ()
                      n742 = call "XYVoltage.vi"("Ring"=w1613) -> ("Y Voltage 2"=w1612:dbl)  [unwired: 7 in, 2 out]
                      n743 = call "XYVoltage.vi"("X Voltage"=w1611, "Y Voltage"=w1612, "Ring"=w1610) -> ()  [unwired: 5 in, 3 out]
                    }
                  }
                }
              }
              frame True {
                n744 = local write "Actual output Amplitude (V)"(w1634) -> ()
                n745 = call "Gen_Square_0to10V.vi"("sampling info"=w1625, "error in (no error)"=w1632, "Width (ms)"=w1635, "amplitude"=w1634, "frequency"=w1633) -> ("error out"=w1620:errorcluster, "signal out"=w1617:waveform(dbl))  [unwired: 5 in]
                n746 = property on="Actual X Output (V)" class="DigNum (strict)"("Blinking"=TRUE) -> ()  [unwired: 2 in, 2 out]
                n747 = local write "Output waveform"(w1617) -> ()
                n748 = call "scale xy steering.vi"("-2.5 to 2.5 V input"=w1615) -> ("0 to 9 V output"=w1614:dbl)  [unwired: 1 in, 1 out]
                n749 = local write "Actual X Output (V)"(w1614) -> ()
                n750 = Initialize Array(w1614, w1628) -> (w1624:dbl[])
                n751 = Bundle By Name("Y"=w1624, "dt"=w1627) -> (w1618:waveform(dbl))  [unwired: 1 in]
                n752 = Merge Signals(w1617, w1630, w1618, w1629, w1626) -> (w1621:dynamicdata)
                n753 = call-poly <vilib>:"DAQmx Write.vi"("task/channels in"=w1631, "data"=w1621, "error in"=w1620) -> ("task out"=w1623:refnum<k21>, "error out"=w1622:errorcluster)  [unwired: 10 in, 1 out]
              }
            }
            n754 = Equal To 0?(x=w1514) -> (x = 0?=w1520:bool)
            n755 = Not(x=w1518) -> (.not. x?=w1521:bool)
            n756 = Or(x=w1521, y=w1520) -> (x .or. y?=w1519:bool)
            n757 = Select(t=w1515, s=w1519, f=w1517) -> (s? t:f=w1516:dbl)
          }
          event "Y Voltage": Value Change {
            w1659 = 0.05 ("y")
            n758 = event-data() -> ("NewVal"=w1637:dbl)  [unwired: 1 in, 4 out]
            n759 = local write "Actual X Output (V)"(w1669) -> ()
            n760 = local write "Actual Needle Output (V)"(w1664) -> ()
            n761 = local write "Actual Einzel Output (V)"(w1673) -> ()
            n762 = Greater?(x=w1637, y=w1650) -> (0:w1661:bool)
            n763 = Subtract(x=w1637, y=w1650) -> (x-y=w1657:dbl)
            n764 = Subtract(x=w1650, y=w1637) -> (x-y=w1658:dbl)
            n765 = Initialize Array(w1669, w1667) -> (w1671:dbl[])
            n766 = Initialize Array(w1664, w1667) -> (w1665:dbl[])
            n767 = Initialize Array(w1673, w1667) -> (w1674:dbl[])
            n768 = Greater?(x=w1657, y=w1658) -> (0:w1660:bool)
            n769 = Bundle By Name("Y"=w1671, "dt"=w1666) -> (w1670:waveform(dbl))  [unwired: 1 in]
            n770 = Bundle By Name("Y"=w1665, "dt"=w1666) -> (w1663:waveform(dbl))  [unwired: 1 in]
            n771 = Bundle By Name("Y"=w1674, "dt"=w1666) -> (w1672:waveform(dbl))  [unwired: 1 in]
            n772 = Select(t=w1657, s=w1660, f=w1658) -> (s? t:f=w1656:dbl)
            n773 = local read "Calibrate XY"() -> (w1654:bool)
            n774 = Divide(x=w1656, y=w1659) -> (x/y=w1655:dbl)
            n775 = To Long Integer(number=w1655) -> (32bit integer=w1636:i32)
            n776 = Or(x=w1654, y=w1652) -> (x .or. y?=w1653:bool)
            n777 = case shown="False" w1653 {
              tunnel: [w1699 w1744] -> w1680
              tunnel: w1679 -> [w1698 w1757]
              tunnel: w1651 -> [w1697 w1756]
              tunnel: w1678 -> [w1696 w1755]
              tunnel: w1677 -> [w1695 w1754]
              tunnel: w1676 -> [w1694 w1753]
              tunnel: [w1693 w1745] -> w1675
              tunnel: w1672 -> [w1692 w1752]
              tunnel: w1670 -> [w1691 w1751]
              tunnel: w1667 -> [w1690 w1750]
              tunnel: w1666 -> [w1689 w1749]
              tunnel: w1663 -> [w1688 w1748]
              tunnel: w1662 -> [w1687 w1747]
              tunnel: w1661 -> [w1686 _]
              tunnel: w1659 -> [w1685 _]
              tunnel: w1636 -> [w1684 _]
              tunnel: w1650 -> [w1683 _]
              tunnel: w1637 -> [_ w1736]
              tunnel: [w1682 w1737] -> w1639
              tunnel: [w1681 FALSE ("Abort Change")] -> w1640
              frame False {
                n778 = for {
                  N: w1684 -> [_]
                  tunnel: w1685 -> [w1729]
                  tunnel: w1683 -> [w1728]
                  tunnel: w1689 -> [w1726]
                  tunnel: w1690 -> [w1725]
                  tunnel: [w1724] -> w1699
                  tunnel: w1698 -> [w1705]
                  tunnel: w1697 -> [w1706]
                  tunnel: w1696 -> [w1720]
                  tunnel: w1695 -> [w1719]
                  tunnel: w1692 -> [w1708]
                  tunnel: w1691 -> [w1716]
                  tunnel: w1688 -> [w1714]
                  shift-right: [w1723] -> w1693
                  shift-left: w1694 -> [w1718]
                  tunnel: w1686 -> [w1710]
                  tunnel: w1687 -> [w1709]
                  tunnel: [w1701] -> w1682
                  tunnel: [w1703] -> w1681
                  i -> [w1730]
                  stop <- w1703 stop-if-true
                  n779 = local write "Actual output Amplitude (V)"(w1706) -> ()
                  n780 = call "Gen_Square_0to10V.vi"("sampling info"=w1709, "error in (no error)"=w1719, "Width (ms)"=w1705, "amplitude"=w1706, "frequency"=w1720) -> ("error out"=w1721:errorcluster, "signal out"=w1707:waveform(dbl))  [unwired: 5 in]
                  n781 = Increment(x=w1730) -> (x+1=w1731:i32)
                  n782 = property on="Actual Y Output (V)" class="DigNum (strict)"("Blinking"=TRUE) -> ()  [unwired: 2 in, 2 out]
                  n783 = local write "Output waveform"(w1707) -> ()
                  n784 = Multiply(x=w1729, y=w1731) -> (x*y=w1712:dbl)
                  n785 = Negate(x=w1712) -> (-x=w1713:dbl)
                  n786 = Select(t=w1712, s=w1710, f=w1713) -> (s? t:f=w1711:dbl)
                  n787 = Add(x=w1728, y=w1711) -> (x+y=w1701:dbl)
                  n788 = call "scale xy steering.vi"("-2.5 to 2.5 V input"=w1701) -> ("0 to 9 V output"=w1700:dbl)  [unwired: 1 in, 1 out]
                  n789 = local write "Actual Y Output (V)"(w1700) -> ()
                  n790 = Initialize Array(w1700, w1725) -> (w1727:dbl[])
                  n791 = Bundle By Name("Y"=w1727, "dt"=w1726) -> (w1715:waveform(dbl))  [unwired: 1 in]
                  n792 = Merge Signals(w1707, w1708, w1716, w1715, w1714) -> (w1722:dynamicdata)
                  n793 = local read "Abort Change"() -> (w1704:bool)
                  n794 = local read "stop"() -> (w1702:bool)
                  n795 = call-poly <vilib>:"DAQmx Write.vi"("task/channels in"=w1718, "data"=w1722, "error in"=w1721) -> ("task out"=w1723:refnum<k21>, "error out"=w1724:errorcluster)  [unwired: 10 in, 1 out]
                  n796 = Or(x=w1704, y=w1702) -> (x .or. y?=w1703:bool)
                  n797 = case shown="True" w1703 {
                    tunnel: w1701 -> [_ w1733]
                    frame False {
                    }
                    frame True {
                      w1732 = T5 4 items=["Get", "Set X", "Set Y", "Set XY", "Internal"] ("Ring")
                      w1735 = T5 0 items=["Get", "Set X", "Set Y", "Set XY", "Internal"] ("Ring")
                      n798 = local write "Y Voltage"(w1733) -> ()
                      n799 = call "XYVoltage.vi"("Ring"=w1735) -> ("X Voltage 2"=w1734:dbl)  [unwired: 7 in, 2 out]
                      n800 = call "XYVoltage.vi"("X Voltage"=w1734, "Y Voltage"=w1733, "Ring"=w1732) -> ()  [unwired: 5 in, 3 out]
                    }
                  }
                }
              }
              frame True {
                n801 = local write "Actual output Amplitude (V)"(w1756) -> ()
                n802 = call "Gen_Square_0to10V.vi"("sampling info"=w1747, "error in (no error)"=w1754, "Width (ms)"=w1757, "amplitude"=w1756, "frequency"=w1755) -> ("error out"=w1742:errorcluster, "signal out"=w1739:waveform(dbl))  [unwired: 5 in]
                n803 = property on="Actual Y Output (V)" class="DigNum (strict)"("Blinking"=TRUE) -> ()  [unwired: 2 in, 2 out]
                n804 = local write "Output waveform"(w1739) -> ()
                n805 = call "scale xy steering.vi"("-2.5 to 2.5 V input"=w1736) -> ("0 to 9 V output"=w1737:dbl)  [unwired: 1 in, 1 out]
                n806 = local write "Actual Y Output (V)"(w1737) -> ()
                n807 = Initialize Array(w1737, w1750) -> (w1746:dbl[])
                n808 = Bundle By Name("Y"=w1746, "dt"=w1749) -> (w1740:waveform(dbl))  [unwired: 1 in]
                n809 = Merge Signals(w1739, w1752, w1751, w1740, w1748) -> (w1743:dynamicdata)
                n810 = call-poly <vilib>:"DAQmx Write.vi"("task/channels in"=w1753, "data"=w1743, "error in"=w1742) -> ("task out"=w1745:refnum<k21>, "error out"=w1744:errorcluster)  [unwired: 10 in, 1 out]
              }
            }
            n811 = Equal To 0?(x=w1636) -> (x = 0?=w1642:bool)
            n812 = Not(x=w1640) -> (.not. x?=w1643:bool)
            n813 = Or(x=w1643, y=w1642) -> (x .or. y?=w1641:bool)
            n814 = Select(t=w1637, s=w1641, f=w1639) -> (s? t:f=w1638:dbl)
          }
          event "Needle Voltage": Value Change {
            (unwired) "needle" ("name (unnamed)")
            w1782 = 0.05 ("y")
            n815 = event-data() -> ("NewVal"=w1759:dbl)  [unwired: 1 in, 4 out]
            n816 = local write "Actual X Output (V)"(w1791) -> ()
            n817 = local write "Actual Y Output (V)"(w1785) -> ()
            n818 = local write "Actual Einzel Output (V)"(w1795) -> ()
            n819 = Greater?(x=w1759, y=w1772) -> (0:w1784:bool)
            n820 = Subtract(x=w1759, y=w1772) -> (x-y=w1778:dbl)
            n821 = Subtract(x=w1772, y=w1759) -> (x-y=w1779:dbl)
            n822 = Initialize Array(w1791, w1789) -> (w1793:dbl[])
            n823 = Initialize Array(w1785, w1789) -> (w1787:dbl[])
            n824 = Initialize Array(w1795, w1789) -> (w1796:dbl[])
            n825 = Greater?(x=w1778, y=w1779) -> (0:w1780:bool)
            n826 = Bundle By Name("Y"=w1793, "dt"=w1788) -> (w1792:waveform(dbl))  [unwired: 1 in]
            n827 = Bundle By Name("Y"=w1787, "dt"=w1788) -> (w1786:waveform(dbl))  [unwired: 1 in]
            n828 = Bundle By Name("Y"=w1796, "dt"=w1788) -> (w1794:waveform(dbl))  [unwired: 1 in]
            n829 = Select(t=w1778, s=w1780, f=w1779) -> (s? t:f=w1777:dbl)
            n830 = Divide(x=w1777, y=w1782) -> (x/y=w1783:dbl)
            n831 = To Long Integer(number=w1783) -> (32bit integer=w1758:i32)
            n832 = for {
              N: w1758 -> [_]
              tunnel: w1782 -> [w1837]
              tunnel: w1772 -> [w1836]
              tunnel: w1788 -> [w1835]
              tunnel: w1789 -> [w1834]
              tunnel: [w1814] -> w1774
              tunnel: w1800 -> [w1812]
              tunnel: w1773 -> [w1813]
              tunnel: w1799 -> [w1830]
              tunnel: w1776 -> [w1829]
              tunnel: w1794 -> [w1826]
              tunnel: w1792 -> [w1818]
              tunnel: w1786 -> [w1825]
              shift-right: [w1833] -> w1797
              shift-left: w1798 -> [w1828]
              tunnel: w1784 -> [w1820]
              tunnel: w1781 -> [w1819]
              tunnel: [w1808] -> w1761
              tunnel: [w1806] -> w1762
              i -> [w1838]
              stop <- w1806 stop-if-true
              n833 = local write "Actual output Amplitude (V)"(w1813) -> ()
              n834 = call "Gen_Square_0to10V.vi"("sampling info"=w1819, "error in (no error)"=w1829, "Width (ms)"=w1812, "amplitude"=w1813, "frequency"=w1830) -> ("error out"=w1831:errorcluster, "signal out"=w1815:waveform(dbl))  [unwired: 5 in]
              n835 = Increment(x=w1838) -> (x+1=w1839:i32)
              n836 = property on="Actual Needle Output (V)" class="DigNum (strict)"("Blinking"=TRUE) -> ()  [unwired: 2 in, 2 out]
              n837 = local write "Output waveform"(w1815) -> ()
              n838 = Multiply(x=w1837, y=w1839) -> (x*y=w1822:dbl)
              n839 = Negate(x=w1822) -> (-x=w1823:dbl)
              n840 = Select(t=w1822, s=w1820, f=w1823) -> (s? t:f=w1821:dbl)
              n841 = Add(x=w1836, y=w1821) -> (x+y=w1817:dbl)
              n842 = Divide(x=w1817, y=1.0) -> (x/y=w1810:dbl)
              n843 = Less Than 0?(x=w1810) -> (x < 0?=w1811:bool)
              n844 = Select(t=0.0, s=w1811, f=w1810) -> (s? t:f=w1808:dbl)
              n845 = local write "Actual Needle Output (V)"(w1808) -> ()
              n846 = Initialize Array(w1808, w1834) -> (w1803:dbl[])
              n847 = In Range and Coerce(upper limit=10.0, x=w1803, lower limit=0.0) -> (coerced(x)=w1802:dbl[])  [unwired: 1 out]
              n848 = Bundle By Name("Y"=w1802, "dt"=w1835) -> (w1824:waveform(dbl))  [unwired: 1 in]
              n849 = Merge Signals(w1815, w1826, w1818, w1825, w1824) -> (w1832:dynamicdata)
              n850 = local read "Abort Change"() -> (w1807:bool)
              n851 = local read "stop"() -> (w1805:bool)
              n852 = call-poly <vilib>:"DAQmx Write.vi"("task/channels in"=w1828, "data"=w1832, "error in"=w1831) -> ("task out"=w1833:refnum<k21>, "error out"=w1814:errorcluster)  [unwired: 10 in, 1 out]
              n853 = Or(x=w1807, y=w1805) -> (x .or. y?=w1806:bool)
              n854 = case shown="True" w1806 {
                tunnel: w1808 -> [_ w1840]
                frame False {
                }
                frame True {
                  n855 = local write "Needle Voltage"(w1840) -> ()
                }
              }
            }
            n856 = Equal To 0?(x=w1758) -> (x = 0?=w1764:bool)
            n857 = Not(x=w1762) -> (.not. x?=w1765:bool)
            n858 = Merge Errors(w1774) -> (w1775:errorcluster)
            n859 = Or(x=w1765, y=w1764) -> (x .or. y?=w1763:bool)
            n860 = Select(t=w1759, s=w1763, f=w1761) -> (s? t:f=w1760:dbl)
          }
          event "stop": Value Change {
            w1854 = 0.0 ("Width (ms) : 3.5")
            w1857 = TRUE ("Blinking")
            n861 = event-data() -> ()  [unwired: 1 in, 1 out]
            n862 = property on="Actual Y Output (V)" class="DigNum (strict)"("Blinking"=w1857) -> ()  [unwired: 2 in, 2 out]
            n863 = property on="Actual Needle Output (V)" class="DigNum (strict)"("Blinking"=w1857) -> ()  [unwired: 2 in, 2 out]
            n864 = property on="Actual output Amplitude (V)" class="DigNum (strict)"("Blinking"=w1857) -> ()  [unwired: 2 in, 2 out]
            n865 = property on="Actual X Output (V)" class="DigNum (strict)"("Blinking"=w1857) -> ()  [unwired: 2 in, 2 out]
            n866 = property on="Actual Einzel Output (V)" class="DigNum (strict)"("Blinking"=w1857) -> ()  [unwired: 2 in, 2 out]
            n867 = Build Array(w1847, w1846) -> (w1845:dbl[])
            n868 = Equal To 0?(x=w1845) -> (x = 0?=w1844:bool[])
            n869 = Or Array Elements(Boolean array=w1844) -> (logical OR=w1843:bool)
            n870 = Not(x=w1843) -> (.not. x?=w1842:bool)
            n871 = Select(t=w1853, s=w1842, f=0.0) -> (s? t:f=w1849:dbl)
            n872 = Greater?(x=w1849, y=w1848) -> (0:w1867:bool)
            n873 = Select(t=w1849, s=w1867, f=w1848) -> (s? t:f=w1858:dbl)
            n874 = Greater?(x=w1852, y=w1858) -> (0:w1861:bool)
            n875 = Select(t=w1852, s=w1861, f=w1858) -> (s? t:f=w1855:dbl)
            n876 = Multiply(x=20.0, y=w1855) -> (x*y=w1851:dbl)
            n877 = Increment(x=w1851) -> (x+1=w1856:dbl)
            n878 = for {
              N: w1856 -> [w1877]
              tunnel: w1846 -> [w1891]
              tunnel: w1847 -> [w1890]
              tunnel: w1869 -> [w1884]
              tunnel: w1853 -> [w1892]
              tunnel: w1865 -> [w1881]
              tunnel: w1866 -> [w1880]
              tunnel: w1848 -> [w1882]
              tunnel: [w1880] -> _ mode=indexing
              shift-right: [w1886] -> w1860
              shift-left: w1868 -> [w1885]
              tunnel: w1852 -> [w1873]
              tunnel: w1863 -> [w1888]
              tunnel: [w1889] -> w1864
              i -> [w1879]
              n879 = Subtract(x=w1877, y=1) -> (x-y=w1876:i32)
              n880 = Wait (ms)(milliseconds to wait=u32 250) -> ()  [unwired: 1 out]
              n881 = Equal?(x=w1876, y=w1879) -> (x = y?=w1878:bool)
              n882 = case shown="False" w1878 {
                tunnel: w1892 -> [w1932 _]
                tunnel: w1891 -> [w1931 _]
                tunnel: w1890 -> [w1930 _]
                tunnel: [w1929 w1940] -> w1887
                tunnel: w1885 -> [w1928 w1940]
                tunnel: w1884 -> [w1924 _]
                tunnel: [w1923 w1941] -> w1883
                tunnel: w1882 -> [w1919 _]
                tunnel: w1877 -> [w1911 _]
                tunnel: w1881 -> [w1907 w1937]
                tunnel: w1880 -> [w1909 w1938]
                tunnel: w1879 -> [w1899 _]
                tunnel: w1873 -> [w1910 _]
                tunnel: [w1901 w1939] -> w1872
                frame False {
                  w1897 = T5 4 items=["Get", "Set X", "Set Y", "Set XY", "Internal"] ("Ring")
                  w1898 = 0.0 ("t")
                  w1906 = 1.0 ("y")
                  n883 = Divide(x=w1919, y=w1911) -> (x/y=w1921:dbl)
                  n884 = Divide(x=w1910, y=w1911) -> (x/y=w1913:dbl)
                  n885 = Divide(x=w1932, y=w1911) -> (x/y=w1927:dbl)
                  n886 = call "XYVoltage.vi"("X Voltage"=w1898, "Y Voltage"=w1898, "Ring"=w1897) -> ("X Voltage 2"=w1895:dbl, "Y Voltage 2"=w1894:dbl)  [unwired: 5 in, 1 out]
                  n887 = Multiply(x=w1921, y=w1899) -> (x*y=w1920:dbl)
                  n888 = Multiply(x=w1913, y=w1899) -> (x*y=w1912:dbl)
                  n889 = Multiply(x=w1927, y=w1899) -> (x*y=w1926:dbl)
                  n890 = call "scale xy steering.vi"("-2.5 to 2.5 V input"=w1894) -> ("0 to 9 V output"=w1893:dbl)  [unwired: 1 in, 1 out]
                  n891 = call "scale xy steering.vi"("-2.5 to 2.5 V input"=w1895) -> ("0 to 9 V output"=w1896:dbl)  [unwired: 1 in, 1 out]
                  n892 = local write "Actual X Output (V)"(w1896) -> ()
                  n893 = local write "Actual Y Output (V)"(w1893) -> ()
                  n894 = Subtract(x=w1919, y=w1920) -> (x-y=w1902:dbl)
                  n895 = Subtract(x=w1910, y=w1912) -> (x-y=w1904:dbl)
                  n896 = Subtract(x=w1932, y=w1926) -> (x-y=w1925:dbl)
                  n897 = Initialize Array(w1896, w1907) -> (w1917:dbl[])
                  n898 = Initialize Array(w1893, w1907) -> (w1915:dbl[])
                  n899 = local write "Actual output Amplitude (V)"(w1925) -> ()
                  n900 = call "Gen_Square_0to10V.vi"("sampling info"=w1924, "error in (no error)"=w1928, "Width (ms)"=w1931, "amplitude"=w1925, "frequency"=w1930) -> ("error out"=w1929:errorcluster, "signal out"=w1901:waveform(dbl))  [unwired: 5 in]
                  n901 = Bundle By Name("Y"=w1917, "dt"=w1909) -> (w1916:waveform(dbl))  [unwired: 1 in]
                  n902 = Bundle By Name("Y"=w1915, "dt"=w1909) -> (w1914:waveform(dbl))  [unwired: 1 in]
                  n903 = Divide(x=w1902, y=w1906) -> (x/y=w1903:dbl)
                  n904 = Divide(x=w1904, y=w1906) -> (x/y=w1905:dbl)
                  n905 = local write "Actual Einzel Output (V)"(w1903) -> ()
                  n906 = local write "Actual Needle Output (V)"(w1905) -> ()
                  n907 = Initialize Array(w1903, w1907) -> (w1922:dbl[])
                  n908 = Initialize Array(w1905, w1907) -> (w1908:dbl[])
                  n909 = Bundle By Name("Y"=w1922, "dt"=w1909) -> (w1918:waveform(dbl))  [unwired: 1 in]
                  n910 = Bundle By Name("Y"=w1908, "dt"=w1909) -> (w1900:waveform(dbl))  [unwired: 1 in]
                  n911 = Merge Signals(w1901, w1918, w1916, w1914, w1900) -> (w1923:dynamicdata)
                }
                frame True {
                  w1934 = 0.0 ("element")
                  n912 = local write "Actual Needle Output (V)"(w1934) -> ()
                  n913 = local write "Needle Voltage"(w1934) -> ()
                  n914 = local write "Desired Amplitude (V)"(w1934) -> ()
                  n915 = local write "Einzel Voltage"(w1934) -> ()
                  n916 = local write "Actual output Amplitude (V)"(w1934) -> ()
                  n917 = local write "X Voltage"(w1934) -> ()
                  n918 = local write "Y Voltage"(w1934) -> ()
                  n919 = local write "Actual Einzel Output (V)"(w1934) -> ()
                  n920 = Initialize Array(w1934, w1937) -> (w1942:dbl[])
                  n921 = call "scale xy steering.vi"("-2.5 to 2.5 V input"=w1934) -> ("0 to 9 V output"=w1933:dbl)  [unwired: 1 in, 1 out]
                  n922 = local write "Actual X Output (V)"(w1933) -> ()
                  n923 = local write "Actual Y Output (V)"(w1933) -> ()
                  n924 = Bundle By Name("Y"=w1942, "dt"=w1938) -> (w1939:waveform(dbl))  [unwired: 1 in]
                  n925 = Initialize Array(w1933, w1937) -> (w1936:dbl[])
                  n926 = Bundle By Name("Y"=w1936, "dt"=w1938) -> (w1935:waveform(dbl))  [unwired: 1 in]
                  n927 = Merge Signals(w1939, w1939, w1935, w1935, w1939) -> (w1941:dynamicdata)
                }
              }
              n928 = local write "Output waveform"(w1872) -> ()
              n929 = call-poly <vilib>:"DAQmx Write.vi"("task/channels in"=w1888, "data"=w1883, "error in"=w1887) -> ("task out"=w1889:refnum<k21>, "error out"=w1886:errorcluster)  [unwired: 10 in, 1 out]
            }
            n930 = flat-sequence {
              tunnel: w1860 -> [w1871]
              tunnel: [w1871] -> w1859
              frame #0 {
                w1870 = TRUE ("Finished")
                n931 = local write "stop"(w1870) -> ()
                "Finished" <- w1870
              }
            }
          }
          event "Desired Amplitude (V)": Value Change {
            w1971 = 0.05 ("y")
            n932 = event-data() -> ("NewVal"=w1950:dbl)  [unwired: 1 in, 1 out]
            n933 = local write "Actual X Output (V)"(w1984) -> ()
            n934 = local write "Actual Needle Output (V)"(w1974) -> ()
            n935 = local write "Actual Einzel Output (V)"(w1987) -> ()
            n936 = Greater?(x=w1950, y=w1963) -> (0:w1973:bool)
            n937 = Subtract(x=w1950, y=w1963) -> (x-y=w1969:dbl)
            n938 = Subtract(x=w1963, y=w1950) -> (x-y=w1967:dbl)
            n939 = Initialize Array(w1984, w1978) -> (w1985:dbl[])
            n940 = Initialize Array(w1982, w1978) -> (w1981:dbl[])
            n941 = Initialize Array(w1974, w1978) -> (w1976:dbl[])
            n942 = Initialize Array(w1987, w1978) -> (w1989:dbl[])
            n943 = Greater?(x=w1969, y=w1967) -> (0:w1970:bool)
            n944 = Bundle By Name("Y"=w1985, "dt"=w1977) -> (w1983:waveform(dbl))  [unwired: 1 in]
            n945 = Bundle By Name("Y"=w1981, "dt"=w1977) -> (w1980:waveform(dbl))  [unwired: 1 in]
            n946 = Bundle By Name("Y"=w1976, "dt"=w1977) -> (w1975:waveform(dbl))  [unwired: 1 in]
            n947 = Bundle By Name("Y"=w1989, "dt"=w1977) -> (w1988:waveform(dbl))  [unwired: 1 in]
            n948 = Select(t=w1969, s=w1970, f=w1967) -> (s? t:f=w1968:dbl)
            n949 = Quotient & Remainder(x=w1968, y=w1971) -> (floor(x/y)=w1972:dbl)  [unwired: 1 out]
            n950 = Build Array(w1948, w1946) -> (w1945:dbl[])
            n951 = Equal To 0?(x=w1945) -> (x = 0?=w1944:bool[])
            n952 = To Long Integer(number=w1972) -> (32bit integer=w1949:i32)
            n953 = Or Array Elements(Boolean array=w1944) -> (logical OR=w1943:bool)
            n954 = case shown="True" w1943 {
              tunnel: w1948 -> [w2010 w2028]
              tunnel: w1946 -> [w2009 w2027]
              tunnel: w1991 -> [w2008 w2026]
              tunnel: w1990 -> [w2007 w2025]
              tunnel: w1988 -> [w2006 w2024]
              tunnel: [w2005 w2023] -> w1986
              tunnel: w1983 -> [w2004 w2022]
              tunnel: w1980 -> [w2003 w2021]
              tunnel: w1975 -> [w2002 w2020]
              tunnel: w1973 -> [_ w2019]
              tunnel: w1971 -> [_ w2018]
              tunnel: w1966 -> [w2001 w2017]
              tunnel: [w2000 w2016] -> w1965
              tunnel: w1963 -> [_ w2015]
              tunnel: [w1999 w2014] -> w1953
              tunnel: [w1992 w2013] -> w1952
              tunnel: w1949 -> [_ w2012]
              tunnel: w1947 -> [w1992 _]
              frame True {
                n955 = property on="Actual output Amplitude (V)" class="DigNum (strict)"("Blinking"=TRUE) -> ()  [unwired: 2 in, 2 out]
                n956 = local write "Actual output Amplitude (V)"(w1992) -> ()
                n957 = call "Gen_Square_0to10V.vi"("sampling info"=w2007, "error in (no error)"=w2001, "Width (ms)"=w2010, "amplitude"=w1992, "frequency"=w2009) -> ("error out"=w1998:errorcluster, "signal out"=w1995:waveform(dbl))  [unwired: 5 in]
                n958 = local write "Output waveform"(w1995) -> ()
                n959 = Merge Signals(w1995, w2006, w2004, w2003, w2002) -> (w1996:dynamicdata)
                n960 = call-poly <vilib>:"DAQmx Write.vi"("task/channels in"=w2008, "data"=w1996, "error in"=w1998) -> ("task out"=w2005:refnum<k21>, "error out"=w2000:errorcluster)  [unwired: 10 in, 1 out]
                n961 = local read "Abort Change"() -> (w1994:bool)
                n962 = local read "stop"() -> (w1993:bool)
                n963 = Or(x=w1994, y=w1993) -> (x .or. y?=w1999:bool)
                n964 = case shown="True" w1999 {
                  tunnel: w1992 -> [_ w2011]
                  frame False {
                  }
                  frame True {
                    n965 = local write "Desired Amplitude (V)"(w2011) -> ()
                  }
                }
              }
              frame False {
                n966 = for {
                  N: w2012 -> [_]
                  tunnel: w2028 -> [w2054]
                  tunnel: w2027 -> [w2053]
                  tunnel: w2015 -> [w2051]
                  tunnel: w2017 -> [w2050]
                  tunnel: [w2048] -> w2016
                  tunnel: w2025 -> [w2046]
                  tunnel: w2018 -> [w2043]
                  tunnel: w2024 -> [w2041]
                  tunnel: w2022 -> [w2039]
                  tunnel: w2021 -> [w2040]
                  tunnel: w2020 -> [w2038]
                  shift-right: [w2047] -> w2023
                  shift-left: w2026 -> [w2049]
                  tunnel: w2019 -> [w2034]
                  tunnel: [w2032] -> w2013
                  tunnel: [w2030] -> w2014
                  i -> [w2052]
                  stop <- w2030 stop-if-true
                  n967 = Increment(x=w2052) -> (x+1=w2045:i32)
                  n968 = property on="Actual output Amplitude (V)" class="DigNum (strict)"("Blinking"=TRUE) -> ()  [unwired: 2 in, 2 out]
                  n969 = Multiply(x=w2043, y=w2045) -> (x*y=w2035:dbl)
                  n970 = Negate(x=w2035) -> (-x=w2037:dbl)
                  n971 = Select(t=w2035, s=w2034, f=w2037) -> (s? t:f=w2036:dbl)
                  n972 = Add(x=w2051, y=w2036) -> (x+y=w2032:dbl)
                  n973 = local write "Actual output Amplitude (V)"(w2032) -> ()
                  n974 = call "Gen_Square_0to10V.vi"("sampling info"=w2046, "error in (no error)"=w2050, "Width (ms)"=w2054, "amplitude"=w2032, "frequency"=w2053) -> ("error out"=w2055:errorcluster, "signal out"=w2033:waveform(dbl))  [unwired: 5 in]
                  n975 = local write "Output waveform"(w2033) -> ()
                  n976 = Merge Signals(w2033, w2041, w2039, w2040, w2038) -> (w2042:dynamicdata)
                  n977 = call-poly <vilib>:"DAQmx Write.vi"("task/channels in"=w2049, "data"=w2042, "error in"=w2055) -> ("task out"=w2047:refnum<k21>, "error out"=w2048:errorcluster)  [unwired: 10 in, 1 out]
                  n978 = local read "Abort Change"() -> (w2031:bool)
                  n979 = local read "stop"() -> (w2029:bool)
                  n980 = Or(x=w2031, y=w2029) -> (x .or. y?=w2030:bool)
                  n981 = case shown="True" w2030 {
                    tunnel: w2032 -> [_ w2056]
                    frame False {
                    }
                    frame True {
                      n982 = local write "Desired Amplitude (V)"(w2056) -> ()
                    }
                  }
                }
              }
            }
            n983 = Equal To 0?(x=w1949) -> (x = 0?=w1955:bool)
            n984 = Not(x=w1953) -> (.not. x?=w1956:bool)
            n985 = Merge Errors(w1965) -> (w1964:errorcluster)
            n986 = Or(x=w1956, y=w1955) -> (x .or. y?=w1954:bool)
            n987 = Select(t=w1950, s=w1954, f=w1952) -> (s? t:f=w1951:dbl)
          }
          event "Frequency": Value Change {
            w2084 = 0.5 ("y")
            n988 = event-data() -> ("NewVal"=w2064:dbl)  [unwired: 1 in, 1 out]
            n989 = local write "Actual X Output (V)"(w2097) -> ()
            n990 = local write "Actual Needle Output (V)"(w2087) -> ()
            n991 = local write "Actual Einzel Output (V)"(w2100) -> ()
            n992 = Greater?(x=w2064, y=w2076) -> (0:w2086:bool)
            n993 = Subtract(x=w2064, y=w2076) -> (x-y=w2082:dbl)
            n994 = Subtract(x=w2076, y=w2064) -> (x-y=w2080:dbl)
            n995 = Initialize Array(w2097, w2091) -> (w2098:dbl[])
            n996 = Initialize Array(w2095, w2091) -> (w2094:dbl[])
            n997 = Initialize Array(w2087, w2091) -> (w2089:dbl[])
            n998 = Initialize Array(w2100, w2091) -> (w2102:dbl[])
            n999 = Greater?(x=w2082, y=w2080) -> (0:w2083:bool)
            n1000 = Bundle By Name("Y"=w2098, "dt"=w2090) -> (w2096:waveform(dbl))  [unwired: 1 in]
            n1001 = Bundle By Name("Y"=w2094, "dt"=w2090) -> (w2093:waveform(dbl))  [unwired: 1 in]
            n1002 = Bundle By Name("Y"=w2089, "dt"=w2090) -> (w2088:waveform(dbl))  [unwired: 1 in]
            n1003 = Bundle By Name("Y"=w2102, "dt"=w2090) -> (w2101:waveform(dbl))  [unwired: 1 in]
            n1004 = Select(t=w2082, s=w2083, f=w2080) -> (s? t:f=w2081:dbl)
            n1005 = Build Array(w2060, w2061) -> (w2059:dbl[])
            n1006 = Quotient & Remainder(x=w2081, y=w2084) -> (floor(x/y)=w2085:dbl)  [unwired: 1 out]
            n1007 = Equal To 0?(x=w2059) -> (x = 0?=w2058:bool[])
            n1008 = Or Array Elements(Boolean array=w2058) -> (logical OR=w2057:bool)
            n1009 = To Long Integer(number=w2085) -> (32bit integer=w2063:i32)
            n1010 = case shown="False" w2057 {
              tunnel: w2060 -> [w2124 w2143]
              tunnel: w2105 -> [w2106 w2142]
              tunnel: w2104 -> [w2123 w2141]
              tunnel: w2103 -> [w2122 w2140]
              tunnel: w2101 -> [w2121 w2139]
              tunnel: [w2120 w2138] -> w2099
              tunnel: w2096 -> [w2119 w2137]
              tunnel: w2093 -> [w2118 w2136]
              tunnel: w2088 -> [w2117 w2135]
              tunnel: w2086 -> [_ w2134]
              tunnel: w2084 -> [_ w2133]
              tunnel: w2079 -> [w2116 w2132]
              tunnel: [w2115 w2131] -> w2078
              tunnel: w2061 -> [w2114 w2130]
              tunnel: w2076 -> [_ w2129]
              tunnel: [w2113 w2128] -> w2066
              tunnel: [w2106 w2127] -> w2065
              tunnel: w2063 -> [_ w2126]
              frame True {
                n1011 = property on="Actual output Frequency" class="DigNum (strict)"("Blinking"=TRUE) -> ()  [unwired: 2 in, 2 out]
                n1012 = call "Gen_Square_0to10V.vi"("sampling info"=w2122, "error in (no error)"=w2116, "Width (ms)"=w2124, "amplitude"=w2114, "frequency"=w2106) -> ("error out"=w2112:errorcluster, "signal out"=w2110:waveform(dbl))  [unwired: 5 in]
                n1013 = local write "Actual output Frequency"(w2106) -> ()
                n1014 = local write "Output waveform"(w2110) -> ()
                n1015 = Merge Signals(w2110, w2121, w2119, w2118, w2117) -> (w2111:dynamicdata)
                n1016 = local read "Abort Change"() -> (w2108:bool)
                n1017 = call-poly <vilib>:"DAQmx Write.vi"("task/channels in"=w2123, "data"=w2111, "error in"=w2112) -> ("task out"=w2120:refnum<k21>, "error out"=w2115:errorcluster)  [unwired: 10 in, 1 out]
                n1018 = local read "stop"() -> (w2107:bool)
                n1019 = Or(x=w2108, y=w2107) -> (x .or. y?=w2113:bool)
                n1020 = case shown="True" w2113 {
                  tunnel: w2106 -> [_ w2125]
                  frame False {
                  }
                  frame True {
                    n1021 = local write "Frequency"(w2125) -> ()
                  }
                }
              }
              frame False {
                n1022 = for {
                  N: w2126 -> [_]
                  tunnel: w2143 -> [w2169]
                  tunnel: w2142 -> [_]
                  tunnel: w2129 -> [w2167]
                  tunnel: w2132 -> [w2166]
                  tunnel: [w2164] -> w2131
                  tunnel: w2140 -> [w2162]
                  tunnel: w2133 -> [w2160]
                  tunnel: w2139 -> [w2158]
                  tunnel: w2137 -> [w2156]
                  tunnel: w2136 -> [w2157]
                  tunnel: w2135 -> [w2155]
                  shift-right: [w2163] -> w2138
                  shift-left: w2141 -> [w2165]
                  tunnel: w2134 -> [w2151]
                  tunnel: w2130 -> [w2148]
                  tunnel: [w2147] -> w2127
                  tunnel: [w2145] -> w2128
                  i -> [w2168]
                  stop <- w2145 stop-if-true
                  n1023 = Increment(x=w2168) -> (x+1=w2161:i32)
                  n1024 = Multiply(x=w2160, y=w2161) -> (x*y=w2152:dbl)
                  n1025 = property on="Actual output Frequency" class="DigNum (strict)"("Blinking"=TRUE) -> ()  [unwired: 2 in, 2 out]
                  n1026 = Negate(x=w2152) -> (-x=w2154:dbl)
                  n1027 = Select(t=w2152, s=w2151, f=w2154) -> (s? t:f=w2153:dbl)
                  n1028 = Add(x=w2167, y=w2153) -> (x+y=w2147:dbl)
                  n1029 = call "Gen_Square_0to10V.vi"("sampling info"=w2162, "error in (no error)"=w2166, "Width (ms)"=w2169, "amplitude"=w2148, "frequency"=w2147) -> ("error out"=w2170:errorcluster, "signal out"=w2150:waveform(dbl))  [unwired: 5 in]
                  n1030 = local write "Actual output Frequency"(w2147) -> ()
                  n1031 = local write "Output waveform"(w2150) -> ()
                  n1032 = Merge Signals(w2150, w2158, w2156, w2157, w2155) -> (w2159:dynamicdata)
                  n1033 = local read "Abort Change"() -> (w2146:bool)
                  n1034 = call-poly <vilib>:"DAQmx Write.vi"("task/channels in"=w2165, "data"=w2159, "error in"=w2170) -> ("task out"=w2163:refnum<k21>, "error out"=w2164:errorcluster)  [unwired: 10 in, 1 out]
                  n1035 = local read "stop"() -> (w2144:bool)
                  n1036 = Or(x=w2146, y=w2144) -> (x .or. y?=w2145:bool)
                  n1037 = case shown="True" w2145 {
                    tunnel: w2147 -> [_ w2171]
                    frame False {
                    }
                    frame True {
                      n1038 = local write "Frequency"(w2171) -> ()
                    }
                  }
                }
              }
            }
            n1039 = Equal To 0?(x=w2063) -> (x = 0?=w2068:bool)
            n1040 = Not(x=w2066) -> (.not. x?=w2069:bool)
            n1041 = Merge Errors(w2078) -> (w2077:errorcluster)
            n1042 = Or(x=w2069, y=w2068) -> (x .or. y?=w2067:bool)
            n1043 = Select(t=w2064, s=w2067, f=w2065) -> (s? t:f=w2062:dbl)
          }
          event "Width (ms) : 0.1": Value Change {
            w2199 = 0.1 ("y")
            n1044 = event-data() -> ("NewVal"=w2177:dbl)  [unwired: 1 in, 1 out]
            n1045 = local write "Actual X Output (V)"(w2212) -> ()
            n1046 = local write "Actual Needle Output (V)"(w2202) -> ()
            n1047 = local write "Actual Einzel Output (V)"(w2215) -> ()
            n1048 = Greater?(x=w2177, y=w2191) -> (0:w2201:bool)
            n1049 = Subtract(x=w2177, y=w2191) -> (x-y=w2197:dbl)
            n1050 = Subtract(x=w2191, y=w2177) -> (x-y=w2195:dbl)
            n1051 = Initialize Array(w2212, w2206) -> (w2213:dbl[])
            n1052 = Initialize Array(w2210, w2206) -> (w2209:dbl[])
            n1053 = Initialize Array(w2202, w2206) -> (w2204:dbl[])
            n1054 = Initialize Array(w2215, w2206) -> (w2217:dbl[])
            n1055 = Greater?(x=w2197, y=w2195) -> (0:w2198:bool)
            n1056 = Bundle By Name("Y"=w2213, "dt"=w2205) -> (w2211:waveform(dbl))  [unwired: 1 in]
            n1057 = Bundle By Name("Y"=w2209, "dt"=w2205) -> (w2208:waveform(dbl))  [unwired: 1 in]
            n1058 = Bundle By Name("Y"=w2204, "dt"=w2205) -> (w2203:waveform(dbl))  [unwired: 1 in]
            n1059 = Bundle By Name("Y"=w2217, "dt"=w2205) -> (w2216:waveform(dbl))  [unwired: 1 in]
            n1060 = Select(t=w2197, s=w2198, f=w2195) -> (s? t:f=w2196:dbl)
            n1061 = Build Array(w2176, w2175) -> (w2174:dbl[])
            n1062 = Quotient & Remainder(x=w2196, y=w2199) -> (floor(x/y)=w2200:dbl)  [unwired: 1 out]
            n1063 = Equal To 0?(x=w2174) -> (x = 0?=w2173:bool[])
            n1064 = Or Array Elements(Boolean array=w2173) -> (logical OR=w2172:bool)
            n1065 = To Long Integer(number=w2200) -> (32bit integer=w2181:i32)
            n1066 = case shown="True" w2172 {
              tunnel: w2220 -> [w2221 w2258]
              tunnel: w2176 -> [w2239 w2257]
              tunnel: w2219 -> [w2238 w2256]
              tunnel: w2218 -> [w2237 w2255]
              tunnel: w2216 -> [w2236 w2254]
              tunnel: [w2235 w2253] -> w2214
              tunnel: w2211 -> [w2234 w2252]
              tunnel: w2208 -> [w2233 w2251]
              tunnel: w2203 -> [w2232 w2250]
              tunnel: w2201 -> [_ w2249]
              tunnel: w2199 -> [_ w2248]
              tunnel: w2194 -> [w2231 w2247]
              tunnel: [w2230 w2246] -> w2193
              tunnel: w2175 -> [w2229 w2245]
              tunnel: w2191 -> [_ w2244]
              tunnel: [w2228 w2243] -> w2184
              tunnel: w2181 -> [_ w2242]
              tunnel: [w2221 w2241] -> w2178
              frame True {
                n1067 = property on="Actual output width (ms)" class="DigNum (strict)"("Blinking"=TRUE) -> ()  [unwired: 2 in, 2 out]
                n1068 = call "Gen_Square_0to10V.vi"("sampling info"=w2237, "error in (no error)"=w2231, "Width (ms)"=w2221, "amplitude"=w2229, "frequency"=w2239) -> ("error out"=w2227:errorcluster, "signal out"=w2225:waveform(dbl))  [unwired: 5 in]
                n1069 = local write "Actual output width (ms)"(w2221) -> ()
                n1070 = local write "Output waveform"(w2225) -> ()
                n1071 = Merge Signals(w2225, w2236, w2234, w2233, w2232) -> (w2226:dynamicdata)
                n1072 = local read "Abort Change"() -> (w2223:bool)
                n1073 = call-poly <vilib>:"DAQmx Write.vi"("task/channels in"=w2238, "data"=w2226, "error in"=w2227) -> ("task out"=w2235:refnum<k21>, "error out"=w2230:errorcluster)  [unwired: 10 in, 1 out]
                n1074 = local read "stop"() -> (w2222:bool)
                n1075 = Or(x=w2222, y=w2223) -> (x .or. y?=w2228:bool)
                n1076 = case shown="True" w2228 {
                  tunnel: w2221 -> [_ w2240]
                  frame False {
                  }
                  frame True {
                    n1077 = local write "Width (ms) : 0.1"(w2240) -> ()
                  }
                }
              }
              frame False {
                n1078 = for {
                  N: w2242 -> [_]
                  tunnel: w2258 -> [_]
                  tunnel: w2257 -> [w2284]
                  tunnel: w2244 -> [w2282]
                  tunnel: w2247 -> [w2281]
                  tunnel: [w2279] -> w2246
                  tunnel: w2255 -> [w2277]
                  tunnel: w2248 -> [w2275]
                  tunnel: w2254 -> [w2273]
                  tunnel: w2252 -> [w2271]
                  tunnel: w2251 -> [w2272]
                  tunnel: w2250 -> [w2270]
                  shift-right: [w2278] -> w2253
                  shift-left: w2256 -> [w2280]
                  tunnel: w2249 -> [w2266]
                  tunnel: w2245 -> [w2264]
                  tunnel: [w2262] -> w2241
                  tunnel: [w2260] -> w2243
                  i -> [w2283]
                  stop <- w2260 stop-if-true
                  n1079 = Increment(x=w2283) -> (x+1=w2276:i32)
                  n1080 = Multiply(x=w2275, y=w2276) -> (x*y=w2267:dbl)
                  n1081 = property on="Actual output width (ms)" class="DigNum (strict)"("Blinking"=TRUE) -> ()  [unwired: 2 in, 2 out]
                  n1082 = Negate(x=w2267) -> (-x=w2269:dbl)
                  n1083 = Select(t=w2267, s=w2266, f=w2269) -> (s? t:f=w2268:dbl)
                  n1084 = Add(x=w2282, y=w2268) -> (x+y=w2262:dbl)
                  n1085 = call "Gen_Square_0to10V.vi"("sampling info"=w2277, "error in (no error)"=w2281, "Width (ms)"=w2262, "amplitude"=w2264, "frequency"=w2284) -> ("error out"=w2285:errorcluster, "signal out"=w2265:waveform(dbl))  [unwired: 5 in]
                  n1086 = local write "Actual output width (ms)"(w2262) -> ()
                  n1087 = local write "Output waveform"(w2265) -> ()
                  n1088 = Merge Signals(w2265, w2273, w2271, w2272, w2270) -> (w2274:dynamicdata)
                  n1089 = local read "Abort Change"() -> (w2261:bool)
                  n1090 = call-poly <vilib>:"DAQmx Write.vi"("task/channels in"=w2280, "data"=w2274, "error in"=w2285) -> ("task out"=w2278:refnum<k21>, "error out"=w2279:errorcluster)  [unwired: 10 in, 1 out]
                  n1091 = local read "stop"() -> (w2259:bool)
                  n1092 = Or(x=w2259, y=w2261) -> (x .or. y?=w2260:bool)
                  n1093 = case shown="True" w2260 {
                    tunnel: w2262 -> [_ w2286]
                    frame False {
                    }
                    frame True {
                      n1094 = local write "Width (ms) : 0.1"(w2286) -> ()
                    }
                  }
                }
              }
            }
            n1095 = Equal To 0?(x=w2181) -> (x = 0?=w2182:bool)
            n1096 = Not(x=w2184) -> (.not. x?=w2183:bool)
            n1097 = Or(x=w2183, y=w2182) -> (x .or. y?=w2180:bool)
            n1098 = Merge Errors(w2193) -> (w2192:errorcluster)
            n1099 = Select(t=w2177, s=w2180, f=w2178) -> (s? t:f=w2179:dbl)
          }
        }
        n1100 = call-poly <userlib>:"Data Changed__ogtk.vi"("Boolean"=w1232) -> ("Changed"=w1233:bool)
        n1101 = And(x=w1255, y=w1232) -> (x .and. y?=w1254:bool)
        n1102 = Or(x=w1254, y=w1233) -> (x .or. y?=w1256:bool)
        n1103 = case shown="True" w1256 {
          tunnel: w1232 -> [_ w1303]
          tunnel: w1258 -> [w1300 w1308]
          tunnel: [w1300 w1307] -> w1257
          tunnel: w1254 -> [_ w1302]
          tunnel: w1231 -> [w1299 w1306]
          tunnel: [w1299 w1305] -> w1230
          frame False {
          }
          frame True {
            n1104 = Select(t=FALSE, s=w1302, f=w1303) -> (s? t:f=w1304:bool)
            n1105 = case shown="False" w1304 {
              tunnel: w1308 -> [w1316 w1320]
              tunnel: [w1309 w1320] -> w1307
              tunnel: w1306 -> [w1314 _]
              tunnel: [w1314 w1318] -> w1305
              frame False {
                n1106 = Get Date/Time In Seconds() -> (seconds since 1Jan1904=w1317:timestamp)
                n1107 = call "LV_to_int_time.vi"("error in (no error)"=w1316, "Time Stamp"=w1317) -> ("error out"=w1312:errorcluster, "Integer Time"=w1315:i64)  [unwired: 7 in]
                n1108 = call "last_exp_settings_query.vi"("error in (no error)"=w1312) -> ("error out"=w1310:errorcluster, "Experiment ID"=w1313:i64)  [unwired: 5 in, 4 out]
                n1109 = Bundle("Integer Time"=w1314, "Integer Time"=w1315, "Experiment ID"=w1313) -> (w1311:T12)  [unwired: 1 in]
                n1110 = call-poly "post_to_db.vi"("error in (no error)"=w1310, "run_times"=w1311) -> ("error out"=w1309:errorcluster)  [unwired: 9 in]
              }
              frame True {
                n1111 = Get Date/Time In Seconds() -> (seconds since 1Jan1904=w1319:timestamp)
                n1112 = call "LV_to_int_time.vi"("Time Stamp"=w1319) -> ("Integer Time"=w1318:i64)  [unwired: 8 in, 1 out]
              }
            }
          }
        }
        n1113 = Unbundle By Name(w1257) -> ("status"=w1226:bool)
        n1114 = local read "Testing"() -> (w1227:bool)
        n1115 = call <vilib>:"Simple Error Handler.vi"("type of dialog (OK msg:1)"=w1285, "error in (no error)"=w1257) -> ("error?"=w1229:bool, "error out"=w1286:errorcluster)  [unwired: 3 in, 3 out]
        n1116 = Not(x=w1227) -> (.not. x?=w1224:bool)
        n1117 = And(x=w1224, y=w1229) -> (x .and. y?=→"error?":bool)
        n1118 = And(x=w1226, y=w1224) -> (x .and. y?=w1225:bool)
        n1119 = Or(x=w1225, y=w1255) -> (x .or. y?=w1287:bool)
        "Execution Number:" <- w1294
      }
      n1120 = call <vilib>:"DAQmx Clear Task.vi"("task in"=w61, "error in"=w76) -> ("error out"=w75:errorcluster)  [unwired: 13 in]
      n1121 = call <vilib>:"DAQmx Stop Task.vi"("task/channels in"=w112, "error in"=w111) -> ("task out"=w104:refnum<k21>, "error out"=w103:errorcluster)  [unwired: 12 in]
      n1122 = call <vilib>:"DAQmx Stop Task.vi"("task/channels in"=w110, "error in"=w109) -> ("task out"=w102:refnum<k21>, "error out"=w101:errorcluster)  [unwired: 12 in]
      n1123 = call <vilib>:"DAQmx Stop Task.vi"("task/channels in"=w106, "error in"=w105) -> ("task out"=w98:refnum<k21>, "error out"=w97:errorcluster)  [unwired: 12 in]
      n1124 = call <vilib>:"DAQmx Stop Task.vi"("task/channels in"=w108, "error in"=w107) -> ("task out"=w100:refnum<k21>, "error out"=w99:errorcluster)  [unwired: 12 in]
      n1125 = call <vilib>:"DAQmx Clear Task.vi"("task in"=w104, "error in"=w103) -> ("error out"=w86:errorcluster)  [unwired: 13 in]
      n1126 = call <vilib>:"DAQmx Clear Task.vi"("task in"=w102, "error in"=w101) -> ("error out"=w85:errorcluster)  [unwired: 13 in]
      n1127 = call <vilib>:"DAQmx Clear Task.vi"("task in"=w98, "error in"=w97) -> ("error out"=w83:errorcluster)  [unwired: 13 in]
      n1128 = call <vilib>:"DAQmx Clear Task.vi"("task in"=w100, "error in"=w99) -> ("error out"=w84:errorcluster)  [unwired: 13 in]
      n1129 = Merge Errors(w86, w85, w84, w83, w87) -> (w81:errorcluster)
      n1130 = call <vilib>:"DAQmx Clear Task.vi"("task in"=w131, "error in"=w127) -> ("error out"=w130:errorcluster)  [unwired: 13 in]
      n1131 = call <vilib>:"Simple Error Handler.vi"("type of dialog (OK msg:1)"=w142, "error in (no error)"=w130) -> ("error out"=w129:errorcluster)  [unwired: 3 in, 4 out]
      n1132 = Merge Errors(w129, w81, w75, w82) -> (w45:errorcluster)
    }
    frame Error {
    }
  }
  "error out" <- w43
